vi "Code String Panel.vi"(11 "Code String":refnum<class "Code String LV.lvclass">) -> ()   [LabVIEW 2016, in "Code String LV.lvclass"]
doc: "Code String panel process.\n--------------------\nCopyright (c) 2019 Analog Devices, Inc. All rights reserved.\n\nRedistribution and use in source and binary forms, with or without modification,\nare permitted provided that the following conditions are met:\n - Redistributions of source code must retain the above copyright notice, this\n list of conditions and the following disclaimer.\n - Redistributions in binary form must reproduce the above copyright notice,\n this list of conditions and the following disclaimer in the documentation\n and/or other materials provided with the distribution.\n - Modified versions of the software must be conspicuously marked as such.\n - This software is licensed solely and exclusively for use with\n processors/products manufactured by or for Analog Devices, Inc.\n - This software may not be combined or merged with other code in any manner\n that would cause the software to become subject to terms and conditions\n which differ from those listed here.\n - Neither the name of Analog Devices, Inc. nor the names of its contributors\n may be used to endorse or promote products derived from this software\n without specific prior written permission.\n - The use of this software may or may not infringe the patent rights of one or\n more patent holders. This license does not release you from the requirement\n that you obtain separate licenses from these patent holders to use this\n software.\n\nTHIS SOFTWARE IS PROVIDED BY ANALOG DEVICES, INC. AND CONTRIBUTORS \"AS IS\" AND\nANY EXPRESS OR IMPLIED WARRANTIES, INCLUDING, BUT NOT LIMITED TO,\nNON-INFRINGEMENT, TITLE, MERCHANTABILITY AND FITNESS FOR A PARTICULAR PURPOSE\nARE DISCLAIMED. IN NO EVENT SHALL ANALOG DEVICES, INC. OR CONTRIBUTORS BE LIABLE\nFOR ANY DIRECT, INDIRECT, INCIDENTAL, SPECIAL, EXEMPLARY, PUNITIVE OR\nCONSEQUENTIAL DAMAGES (INCLUDING, BUT NOT LIMITED TO, DAMAGES ARISING OUT OF\nCLAIMS OF INTELLECTUAL PROPERTY RIGHTS INFRINGEMENT; PROCUREMENT OF SUBSTITUTE\nGOODS OR SERVICES; LOSS OF USE, DATA, OR PROFITS; OR BUSINESS INTERRUPTION)\nHOWEVER CAUSED AND ON ANY THEORY OF LIABILITY, WHETHER IN CONTRACT, STRICT\nLIABILITY, OR TORT (INCLUDING NEGLIGENCE OR OTHERWISE) ARISING IN ANY WAY OUT OF\nTHE USE OF THIS SOFTWARE, EVEN IF ADVISED OF THE POSSIBILITY OF SUCH DAMAGE.\n\n2019-01-10-7CBSD SLA"
uses:
  Code String LV.lvclass
  C:/Git/ipn_lv_dev/code-string/source/library/Code String/Code String/Code String.lvclass
  Code String/UI Logic/ASCII.ctl
  Code String/Events/Menu Item.ctl
  Suggestion Box/Suggestion Box.lvclass
  Suggestion Box/Events/Update Data.ctl
  <vilib>/Utility/miscctls.llb/LVPositionTypeDef.ctl
  <vilib>/Utility/miscctls.llb/LVSelectionTypeDef.ctl
  <vilib>/Utility/miscctls.llb/LVPointTypeDef.ctl
  <vilib>/Utility/miscctls.llb/LVRectTypeDef.ctl
  Suggestion Box/Suggestion Box.lvclass/Suggestion Box.ctl
  <vilib>/event_ctls.llb/lveventtype.ctl
  <vilib>/Utility/miscctls.llb/LVFontTypeDef.ctl
  Code String/State/Write Selected Text State.vi
  Code String/Properties/Read Completion.vi
  Code String/Properties/Read Editable.vi
  Code String/Properties/Write Completion.vi
  Code String/State/Write Text State.vi
  Code String/Properties/Read Active Ref.vi
  Code String/Properties/Read User Menu Items.vi
  Code String/Properties/Write User Menu Items.vi
  Code String/Properties/Read Rendezvous.vi
  Code String/Properties/Read User Events.vi
  Code String/Properties/Read Delimiter Pattern.vi
  <userlib>/_OpenG.lib/comparison/comparison.llb/String Changed__ogtk.vi
  Code String/Properties/Write Selected Line(s).vi
  Code String/Properties/Write # Selected Lines.vi
  Code String/Properties/Write Selected Token.vi
  Code String/Properties/Font Global.vi
  Code String/Properties/Write Active Ref.vi
  Code String/Properties/Read Selected Text.vi
  Code String/Properties/Read Text.vi
  <userlib>/_OpenG.lib/comparison/comparison.llb/U32 Changed__ogtk.vi
  Code String/Properties/Read Keywords.vi
  <userlib>/_OpenG.lib/comparison/comparison.llb/I32 Changed__ogtk.vi
  Code String/Code String.lvclass
panel:
  in  "Decoration":string
  in  "Line Numbers":i32(listbox)=-1
  out "String Indicator":string
  in  "String Control":string
  in  "Scrollbar":i32(c297)
  # "Copyright (c) 2019 Analog Devices, Inc.  All rights reserved.\n\nRedistribution and use in source and binary forms, with or without modification,\nare permitted provided that the following conditions are met:\n  - Redistributions of source code must retain the above copyright notice, this\n    list of conditions and the following disclaimer.\n  - Redistributions in binary form must reproduce the above copyright notice,\n    this list of conditions and the following disclaimer in the documentation\n    and/or other materials provided with the distribution.\n  - Modified versions of the software must be conspicuously marked as such.\n  - This software is licensed solely and exclusively for use with\n    processors/products manufactured by or for Analog Devices, Inc.\n  - This software may not be combined or merged with other code in any manner\n    that would cause the software to become subject to terms and conditions\n    which differ from those listed here.\n  - Neither the name of Analog Devices, Inc. nor the names of its contributors\n    may be used to endorse or promote products derived from this software\n    without specific prior written permission.\n  - The use of this software may or may not infringe the patent rights of one or\n    more patent holders.  This license does not release you from the requirement\n    that you obtain separate licenses from these patent holders to use this\n    software.\n\nTHIS SOFTWARE IS PROVIDED BY ANALOG DEVICES, INC. AND CONTRIBUTORS \"AS IS\" AND\nANY EXPRESS OR IMPLIED WARRANTIES, INCLUDING, BUT NOT LIMITED TO,\nNON-INFRINGEMENT, TITLE, MERCHANTABILITY AND FITNESS FOR A PARTICULAR PURPOSE\nARE DISCLAIMED. IN NO EVENT SHALL ANALOG DEVICES, INC. OR CONTRIBUTORS BE LIABLE\nFOR ANY DIRECT, INDIRECT, INCIDENTAL, SPECIAL, EXEMPLARY, PUNITIVE OR\nCONSEQUENTIAL DAMAGES (INCLUDING, BUT NOT LIMITED TO, DAMAGES ARISING OUT OF\nCLAIMS OF INTELLECTUAL PROPERTY RIGHTS INFRINGEMENT; PROCUREMENT OF SUBSTITUTE\nGOODS OR SERVICES; LOSS OF USE, DATA, OR PROFITS; OR BUSINESS INTERRUPTION)\nHOWEVER CAUSED AND ON ANY THEORY OF LIABILITY, WHETHER IN CONTRACT, STRICT\nLIABILITY, OR TORT (INCLUDING NEGLIGENCE OR OTHERWISE) ARISING IN ANY WAY OUT OF\nTHE USE OF THIS SOFTWARE, EVEN IF ADVISED OF THE POSSIBILITY OF SUCH DAMAGE.\n\n2019-01-10-7CBSD SLA"
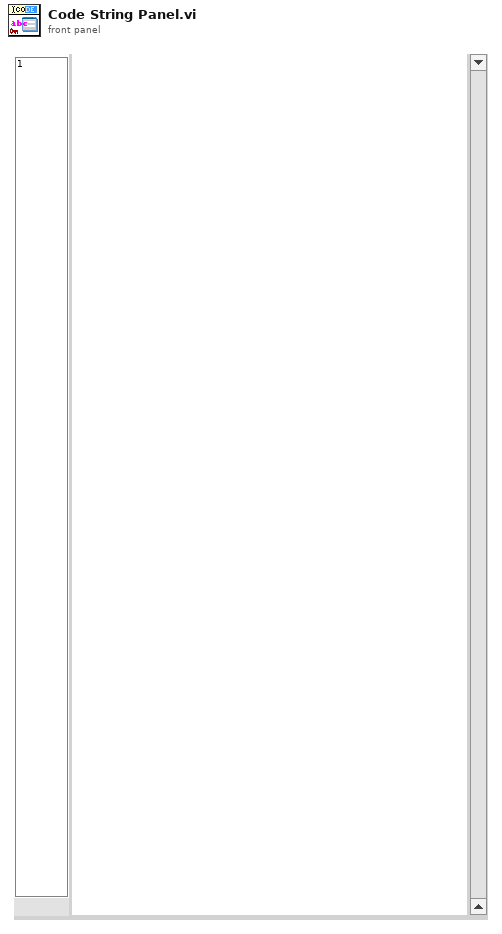
[diagram p1: front panel]
types:
  T1 = typedef "Code String.lvclass/ASCII.ctl" = enum8{"NUL", "SOH", "STX", "ETX", "EOT", "ENQ", "ACK", "BEL", "BS", "HT", "LF", "VT", "FF", "CR", "SO", "SI", "DLE", "DC1", "DC2", "DC3", "DC4", "NAK", "SYN", "ETB", "CAN", "EM", "SUB", "ESC", "FS", "GS", "RS", "US", "SP", "!", "\"", "#", "$", "%", "&", "'", "(", ")", "*", "+", ",", "- ", ".", "/", "0", "1", "2", "3", "4", "5", "6", "7", "8", "9", ":", ";", "<", "=", ">", "?", "@", "A", "B", "C", "D", "E", "F", "G", "H", "I", "J", "K", "L", "M", "N", "O", "P", "Q", "R", "S", "T", "U", "V", "W", "X", "Y", "Z", "[", "\\", "]", "^", "_", "`", "a", "b", "c", "d", "e", "f", "g", "h", "i", "j", "k", "l", "m", "n", "o", "p", "q", "r", "s", "t", "u", "v", "w", "x", "y", "z", "{", "|", "}", "~", "DEL"}
  T2 = typedef "Code String.lvclass/Menu Item.ctl" = cluster{"Item Path":string, "Visible?":bool, "Checked?":bool}
  T3 = enum32{"Invalid", "Standard", "Closed", "Hidden", "Minimized", "Maximized"}
  T4 = enum32{"invalid app kind", "Development System", "Run Time System", "Student Edition", "Embedded LabVIEW", "Evaluation", "Custom"}
  T5 = typedef "lveventtype.ctl" = enum32{"Null", "Timeout", "Annotation Menu Selection", "Annotation Menu Selection?", "App Instance Close", "App Instance Close?", "Autoscale Range Change", "Bookmark Info Change", "Cell Edit", "Cell Edit?", "Cursor Grab", "Cursor Grab?", "Cursor Menu Selection", "Cursor Menu Selection?", "Cursor Move", "Cursor Release", "Data Change", "Direction Change", "Display State Change", "Drag Ended", "Drag Enter", "Drag Leave", "Drag Over", "Drag Source Update", "Drag Starting", "Drag Starting?", "Drop", "Exec State Change", "Key Down", "Key Down?", "Key Repeat", "Key Repeat?", "Key Up", "Listbox Double Click", "Menu Activation?", "Menu Selection (App)", "Menu Selection? (App)", "Menu Selection (User)", "Mouse Down", "Mouse Down?", "Mouse Enter", "Mouse Leave", "Mouse Move", "Mouse Up", "Mouse Wheel", "NI Security User Change (App)", "Pane Size", "Panel Close", "Panel Close?", "Panel Resize", "Plot Attribute Change", "Scale Range Change", "Shortcut Menu Activation?", "Shortcut Menu Selection (App)", "Shortcut Menu Selection? (App)", "Shortcut Menu Selection (User)", "Tree Double Click", "Tree Drag", "Tree Drag?", "Tree Drop", "Tree Drop?", "Tree Item Close", "Tree Item Close?", "Tree Item Open", "Tree Item Open?", "User Event", "Value Change"}
  T6 = typedef "LVPointTypeDef.ctl" = cluster{"Horizontal":i16, "Vertical":i16}
  T7 = cluster{"Selection Start":i32, "Selection End":i32}
  T8 = typedef "LVPositionTypeDef.ctl" = cluster{"Left":i32, "Top":i32}
  T9 = typedef "LVFontTypeDef.ctl" = cluster{"Font Name":string, "Size":u16, "Bold":bool, "Italic":bool, "Underline":bool, "Strikeout":bool, "Color":u32}
  T10 = typedef "LVPoint32TypeDef.ctl" = cluster{"Horizontal":i32, "Vertical":i32}
  T11 = typedef "Suggestion Box.lvclass/Update Data.ctl" = cluster{"Query":string, "Keywords":string[], "Position":T8}
  T12 = typedef "LVSelectionTypeDef.ctl" = cluster{"Selection Start":u32, "Selection End":u32}
  T13 = typedef "LVRectTypeDef.ctl" = cluster{"Left":i16, "Top":i16, "Right":i16, "Bottom":i16}
  T14 = cluster{"Core":cluster{"Current VI Reference":refnum<vi>, "Close Panel on Exit?":bool}, "T":i32, "Panes":refnum<vi>[], "Strings":refnum<vi>[], "Line #":refnum<vi>, "Scrollbar":refnum<vi>, "Suggestions":cluster{"Suggestion Box":refnum<class "Suggestion Box.lvclass">, "Visible?":bool, "Display Limit":i32, "Update Data":T11, "Selected":string, "Location":T12, "Delta?":bool}, "Mouse Down":cluster{"?":bool, "Offset":T6, "Bounds":T13}}
  T15 = typedef "eventvkey.ctl" = enum16{"ASCII", "Enter", "Return", "Shift", "Ctrl", "Alt", "Cmd", "Opt", "Caps", "NumLock", "Clear", "Break", "Up", "Down", "Left", "Right", "Insert", "Delete", "Home", "End", "PageUp", "PageDown", "Escape", "Help", "Pause", "ScrollLock", "F1", "F2", "F3", "F4", "F5", "F6", "F7", "F8", "F9", "F10", "F11", "F12", "F13", "F14", "F15", "F16", "F17", "F18", "F19", "F20", "F21", "F22", "F23", "F24", "Play", "VolumeUp", "VolumeDown", "Mute", "Two Byte Char"}
  T16 = typedef "Rendezvous RefNum" = refnum<k1>
  T17 = cluster{"Suggestion Box":refnum<class "Suggestion Box.lvclass">, "Visible?":bool, "Display Limit":i32, "Update Data":T11, "Selected":string, "Location":T12, "Delta?":bool}
  T18 = cluster{"Current VI Reference":refnum<vi>, "Close Panel on Exit?":bool}
  T19 = typedef "Code String.lvclass/User Events.ctl" = cluster{"Exit":refnum<user-event>, "Editable Changed":refnum<user-event>, "Font Size Changed":refnum<user-event>, "Font Color Changed":refnum<user-event>, "Text Selection Start Changed":refnum<user-event>, "Text Selection End Changed":refnum<user-event>, "Scroll Position Changed":refnum<user-event>, "Shortcut Menu Item":refnum<user-event>, "Text":refnum<user-event>, "Selected Text":refnum<user-event>}
  T20 = typedef "Suggestion Box.lvclass/Public Events.ctl" = cluster{"Suggestion Selected":refnum<user-event>}
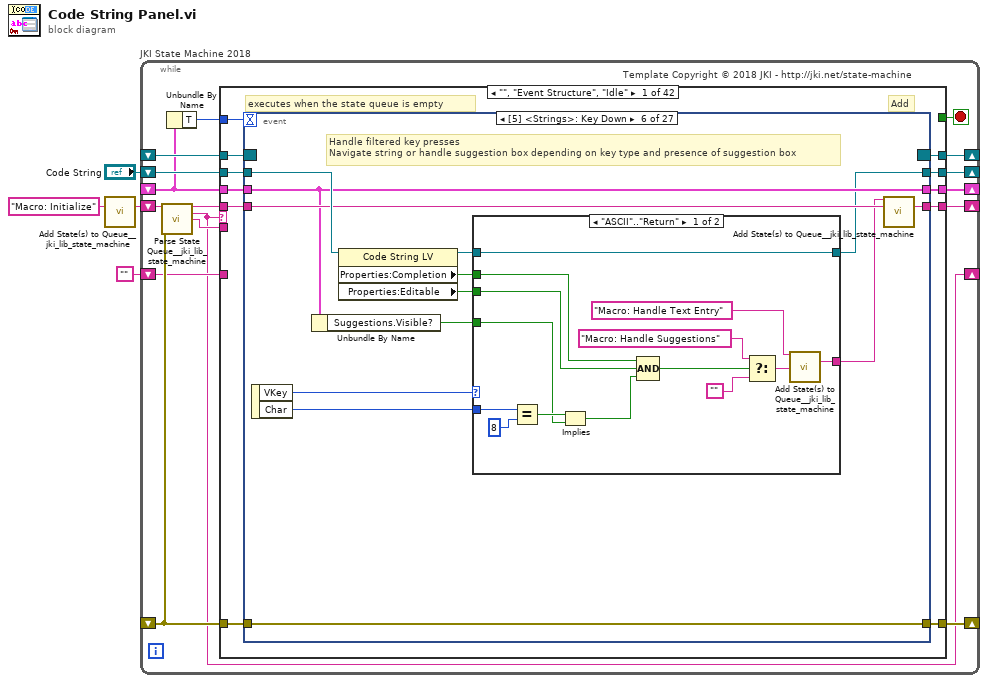
[diagram p0: block diagram]
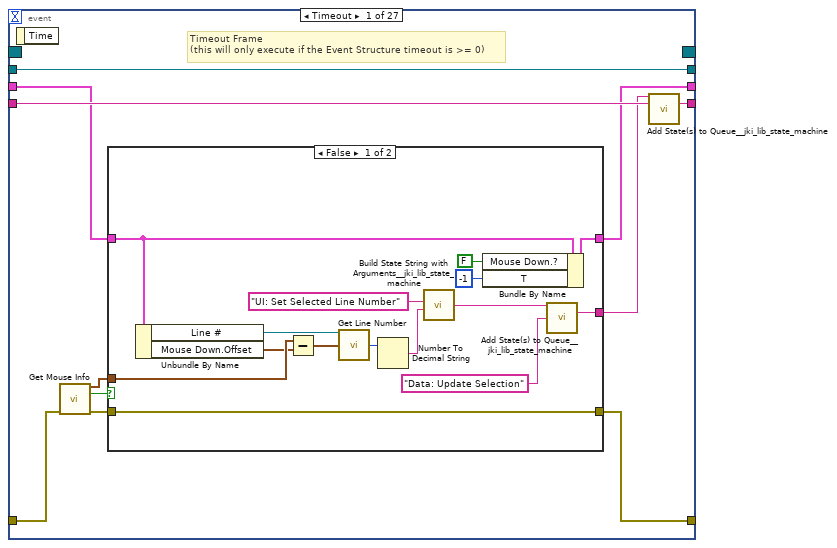
[diagram p2: hidden frame]
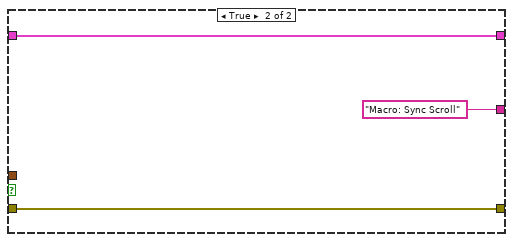
[diagram p3: hidden frame]
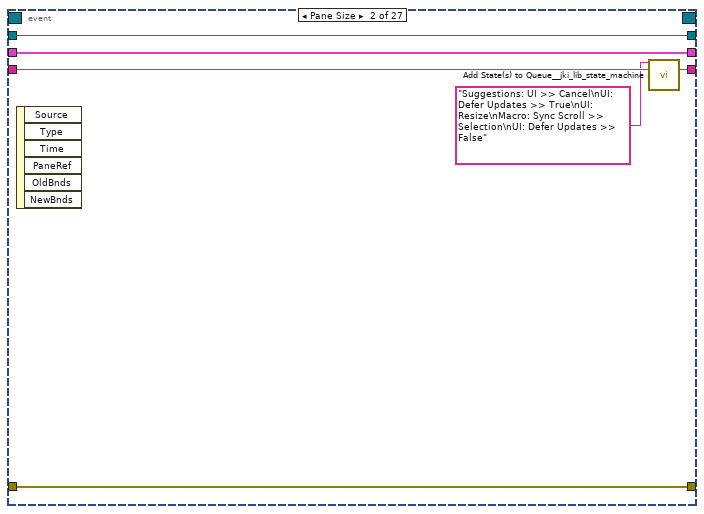
[diagram p4: hidden frame]
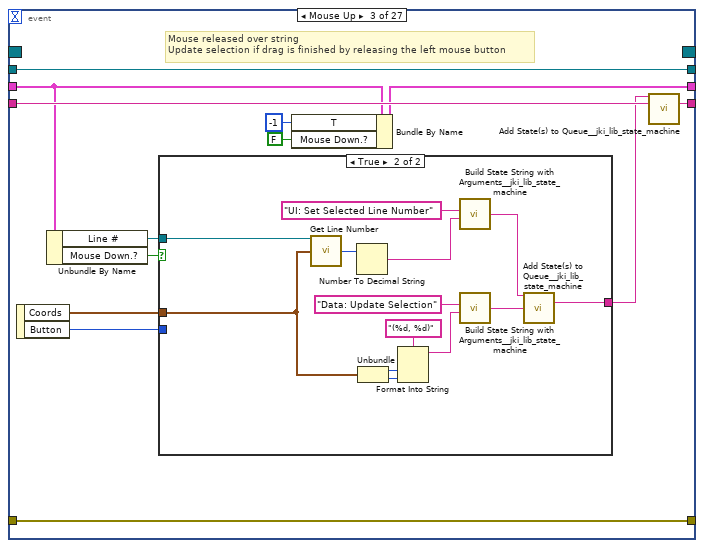
[diagram p5: hidden frame]
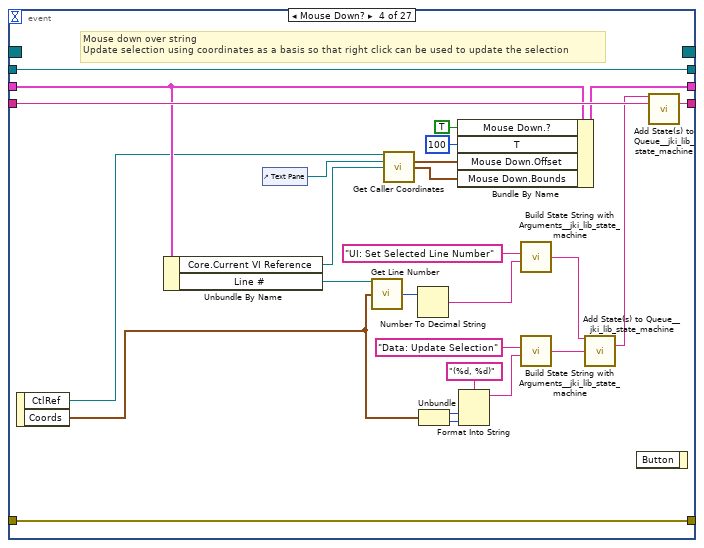
[diagram p7: hidden frame]
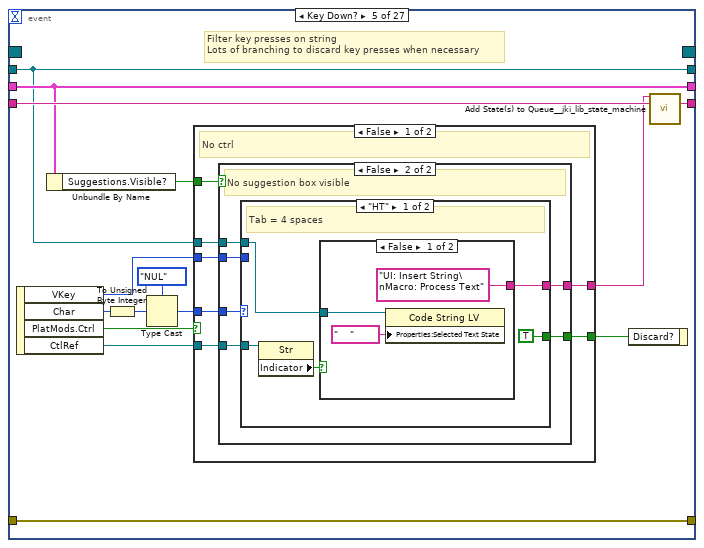
[diagram p8: hidden frame]
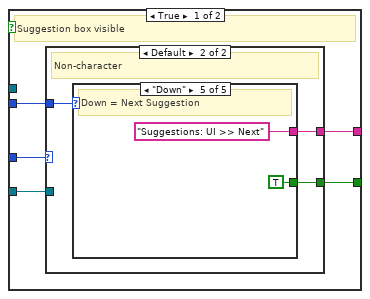
[diagram p9: hidden frame]
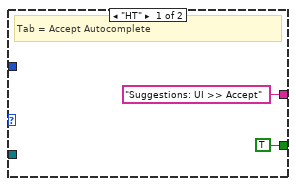
[diagram p10: hidden frame]
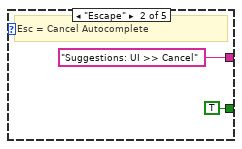
[diagram p12: hidden frame]
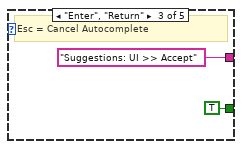
[diagram p13: hidden frame]
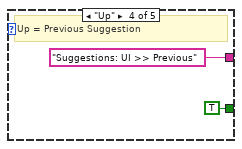
[diagram p14: hidden frame]
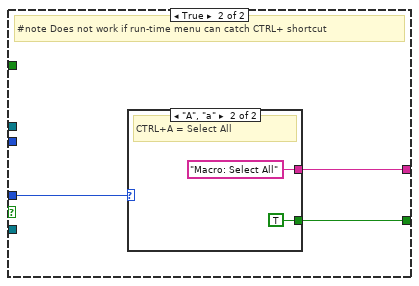
[diagram p17: hidden frame]
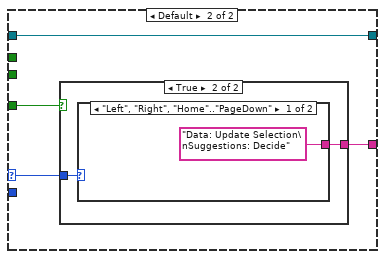
[diagram p19: hidden frame]
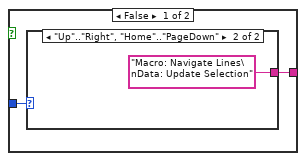
[diagram p20: hidden frame]
diagram:
  n1 = call <vilib>:"Add State(s) to Queue__jki_lib_state_machine.vi"("State(s) in (\"\")"="Macro: Initialize") -> ("States Out"=w4:string)  [unwired: 14 in]
  n2 = while "JKI State Machine 2018" {
    shift-right: [w15] -> _
    shift-left: _ -> [w9]
    shift-right: [w17] -> _
    shift-left: _ -> [w14]
    shift-right: [w8] -> _
    shift-left: w4 -> [w18]
    shift-right: [w13] -> _
    shift-left: "Code String" -> [w12]
    shift-right: [w11] -> _
    shift-left: _ -> [w10]
    shift-right: [w6] -> _
    shift-left: "" -> [w7]
    stop <- w16 stop-if-true
    # "Template Copyright © 2018 JKI - http://jki.net/state-machine"
    n3 = call <vilib>:"Parse State Queue__jki_lib_state_machine.vi"("State Queue"=w18, "Error In (no error)"=w14) -> ("Remaining States"=w20:string, "Current State"=w6:string, "Arguments"=w19:string)  [unwired: 11 in]
    n4 = Unbundle By Name(w9) -> ("T"=w5:i32)
    n5 = case shown="\"\", \"Event Structure\", \"Idle\"" w6 {
      selector: w6 -> [_ _ w480 _ _ _ _ _ _ _ _ _ _ _ _ _ _ _ _ _ _ _ _ _ _ _ _ _ _ _ _ _ _ _ _ _ _ _ _ _ _ _]
      tunnel: w20 -> [w31 w477 w484 w505 w514 w522 w529 w535 w557 w570 w591 w627 w642 w648 w674 w692 w705 w784 w801 w816 w838 w857 w868 w920 w935 w951 w978 w1000 w1024 w1039 w1057 w1073 w1082 w1152 w1159 w1179 w1192 w1199 w1206 w1217 w1235 w1256]
      tunnel: w19 -> [_ _ _ _ _ _ _ _ _ _ w582 _ _ _ _ w687 w699 w780 _ _ w826 _ w864 _ w927 w946 _ w997 _ _ _ _ w1076 _ _ w1172 w1183 _ _ _ w1224 w1242]
      tunnel: w9 -> [w29 w474 w482 w498 w512 w519 w527 w532 _ w567 w588 w625 w637 w645 w650 w690 w701 w779 w787 w815 w834 w849 w859 w910 w929 w944 w967 w992 w1021 w1032 w1041 w1065 w1081 w1149 w1156 w1176 w1189 w1196 w1203 w1220 w1238 w1253]
      tunnel: [w28 w475 w486 w502 w508 errorcluster {"status"=FALSE, "code"=0, "source"=""} ("error out") w526 w533 w555 w568 w581 w617 w638 w646 w666 w688 w702 w771 w799 w810 w836 w851 w865 w918 w933 w949 w976 w993 w1022 w1035 w1045 w1071 w1077 w1150 w1157 w1177 w1190 w1197 w1204 w1221 w1239 w1254] -> w17
      tunnel: w14 -> [w27 w475 w485 w502 w509 w518 w526 w533 w555 w563 w589 w618 w639 w646 w666 w689 w703 w774 w799 w811 w836 w852 w865 w918 w933 w949 w976 w994 w1022 w1035 w1046 w1071 w1078 w1150 w1157 w1177 w1190 w1197 w1204 w1221 w1239 w1254]
      tunnel: [w30 w476 w483 w504 w513 w521 w528 w534 w557 w569 w590 w626 w641 w647 w673 w691 w704 w783 w800 w816 w837 w856 w868 w919 w934 w950 w977 w999 w1023 w1038 w1056 w1072 w1082 w1151 w1158 w1178 w1191 w1198 w1205 w1222 w1240 w1255] -> w8
      tunnel: [_ _ _ _ _ _ TRUE _ _ _ _ _ _ _ _ _ _ _ _ _ _ _ _ _ _ _ _ _ _ _ _ _ _ _ _ _ _ _ _ _ _ _] -> w16
      tunnel: [w26 w474 w482 w503 w512 w519 w527 w532 w556 w567 w575 w625 w637 w645 w650 w690 w701 w779 w787 w815 w834 w849 w859 w910 w929 w944 w967 w992 w1021 w1036 w1053 w1065 w1079 w1149 w1156 w1176 w1189 w1196 w1203 w1220 w1238 w1253] -> w15
      tunnel: w5 -> [w25 _ _ _ _ _ _ _ _ _ _ _ _ _ _ _ _ _ _ _ _ _ _ _ _ _ _ _ _ _ _ _ _ _ _ _ _ _ _ _ _ _]
      tunnel: [w22 w473 w479 w492 w507 w516 w524 w531 w543 w558 w579 w621 w636 w644 w656 w686 w698 w782 w788 w814 w829 w853 w861 w912 w930 w947 w973 w995 w1020 w1034 w1054 w1068 w1074 w1148 w1154 w1170 w1188 w1195 w1202 w1219 w1237 w1247] -> w13
      tunnel: w12 -> [w23 w473 w479 w492 w507 w516 w524 w531 w543 w558 w586 w622 w636 w644 w656 w686 w698 w782 w788 w814 w828 w854 w866 w912 w930 w947 w973 w995 w1020 w1034 w1054 w1068 w1075 w1148 w1154 w1170 w1188 w1195 w1202 w1219 w1237 w1247]
      tunnel: [w24 w472 w478 w491 w511 w515 w523 w530 w553 w562 w587 w619 w634 w643 w672 w685 w697 w781 w798 w812 w835 w855 w867 w917 w932 w948 w975 w998 w1019 w1037 w1055 w1070 w1080 w1147 w1153 w1175 w1187 w1194 w1201 w1218 w1236 w1246] -> w11
      tunnel: w10 -> [w21 w472 w478 w491 w511 w515 w523 w530 w553 _ w587 w620 w634 w643 w672 w685 w697 w781 w798 w813 w835 w855 w867 w917 w932 w948 w975 w998 w1019 w1037 w1055 w1070 w1080 w1147 w1153 w1175 w1187 w1194 w1201 w1218 w1236 w1246]
      tunnel: w7 -> [_ _ _ _ _ _ _ _ _ _ _ _ _ _ _ _ _ _ _ _ _ _ _ _ _ _ _ _ _ _ _ _ _ _ _ _ _ _ _ w1207 w1226 _]
      frame "", "Event Structure", "Idle" {
        # "Add"
        # "executes when the state queue is empty"
        n6 = event shown="[5] <Strings>: Key Down" {
          selector: w21 -> [_ _ _ _ _ _ _ _ _ _ _ _ _ _ _ _ _ _ _ _ _ _ _ _ _ _ _]
          dyn-events: [_ _ _ _ _ _ _ _ _ _ _ _ _ _ _ _ _ _ _ _ _ _ _ _ _ _ _] -> w24
          timeout: w25 -> [_ _ _ _ _ _ _ _ _ _ _ _ _ _ _ _ _ _ _ _ _ _ _ _ _ _ _]
          tunnel: w31 -> [w42 w62 w77 w116 w126 w187 w220 w228 w240 w251 w296 w305 w313 w329 w340 w366 w371 w380 w392 w404 w416 w422 w428 w442 w447 w461 w471]
          tunnel: [w41 w63 w78 w117 w127 w188 w220 w229 w241 w252 w296 w306 w313 w330 w341 w367 w372 w381 w393 w405 w417 w423 w429 w442 w448 w462 w470] -> w30
          tunnel: w29 -> [w33 w66 w73 w100 w124 w183 w219 w225 w244 w254 w294 w303 w311 w322 w348 w369 w375 w384 w396 w408 w419 w425 w431 w434 w452 w464 w468]
          tunnel: [w38 w64 w79 w118 w119 w189 w217 w230 w242 w249 w292 w307 w312 w331 w343 w365 w373 w382 w394 w406 w418 w424 w430 w440 w450 w454 w469] -> w28
          tunnel: w27 -> [w40 w64 w79 w118 w119 w189 w217 w230 w242 w253 w289 w307 w312 w331 w346 w365 w373 w382 w394 w406 w418 w424 w430 w440 w450 w454 w469]
          tunnel: [w32 w66 w70 w108 w124 w183 w219 w225 w244 w254 w294 w303 w311 w322 w348 w369 w375 w384 w396 w408 w419 w425 w431 w434 w449 w464 w468] -> w26
          tunnel: w23 -> [w36 w65 w74 w93 w120 w190 w218 w223 w243 w250 w287 w304 w310 w324 w333 w368 w374 w383 w395 w407 w415 w420 w426 w441 w451 w463 w465]
          tunnel: [w36 w65 w74 w93 w120 w179 w218 w223 w243 w247 w285 w304 w310 w324 w333 w368 w374 w383 w395 w407 w415 w420 w426 w439 w451 w463 w465] -> w22
          event Timeout {
            # "Timeout Frame\n(this will only execute if the Event Structure timeout is >= 0)"
            n7 = event-data() -> ()  [unwired: 1 in, 1 out]
            n8 = call "Get Mouse Info.vi"("error in (no error)"=w40) -> ("Coordinates"=w35:T10, "Left Mouse Button?"=w37:bool, "error out"=w39:errorcluster)  [unwired: 11 in, 1 out]
            n9 = case shown="False" w37 {
              tunnel: w39 -> [w57 w58]
              tunnel: [w57 w58] -> w38
              tunnel: w35 -> [w56 _]
              tunnel: [w45 "Macro: Sync Scroll"] -> w34
              tunnel: w33 -> [w55 w60]
              tunnel: [w43 w60] -> w32
              frame False {
                n10 = Unbundle By Name(w55) -> ("Line #"=w54:refnum<vi>, "Mouse Down.Offset"=w47:T6)
                n11 = Subtract(x=w56, y=w47) -> (x-y=w48:T10)
                n12 = call "Get Line Number.vi"("Line Numbers in"=w54, "Coords"=w48) -> ("Row"=w51:i32)  [unwired: 12 in, 1 out]
                n13 = Number To Decimal String(number=w51) -> (decimal integer string=w52:string)  [unwired: 1 in]
                n14 = call <vilib>:"Build State String with Arguments__jki_lib_state_machine.vi"("Arguments (\"\")"=w52, "State"="UI: Set Selected Line Number") -> ("State with Arguments"=w46:string)  [unwired: 4 in]
                n15 = Bundle By Name(cluster=w55, "Mouse Down.?"=FALSE ("Mouse Down?"), "T"=-1) -> (w43:T14)
                n16 = call <vilib>:"Add State(s) to Queue__jki_lib_state_machine.vi"("State(s) in Front (\"\")"=w46, "State(s) at Back (\"\")"="Data: Update Selection") -> ("States Out"=w45:string)  [unwired: 13 in]
              }
              frame True {
              }
            }
            n17 = call <vilib>:"Add State(s) to Queue__jki_lib_state_machine.vi"("State(s) in Front (\"\")"=w34, "State(s) in (\"\")"=w42) -> ("States Out"=w41:string)  [unwired: 13 in]
          }
          event Pane Size {
            n18 = event-data() -> ()  [unwired: 1 in, 6 out]
            n19 = call <vilib>:"Add State(s) to Queue__jki_lib_state_machine.vi"("State(s) in Front (\"\")"="Suggestions: UI >> Cancel\nUI: Defer Updates >> True\nUI: Resize\nMacro: Sync Scroll >> Selection\nUI: Defer Updates >> False", "State(s) in (\"\")"=w62) -> ("States Out"=w63:string)  [unwired: 13 in]
          }
          event Mouse Up {
            # "Mouse released over string\nUpdate selection if drag is finished by releasing the left mouse button"
            n20 = event-data() -> ("Coords"=w71:T10, "Button"=w76:u16)  [unwired: 1 in]
            n21 = Unbundle By Name(w73) -> ("Line #"=w68:refnum<vi>, "Mouse Down.?"=w72:bool)
            n22 = case shown="True" w72 {
              tunnel: w76 -> [_ _]
              tunnel: [_ w92] -> w75
              tunnel: w71 -> [_ w91]
              tunnel: w68 -> [_ w90]
              frame False {
              }
              frame True {
                n23 = call "Get Line Number.vi"("Line Numbers in"=w90, "Coords"=w91) -> ("Row"=w83:i32)  [unwired: 12 in, 1 out]
                n24 = Number To Decimal String(number=w83) -> (decimal integer string=w84:string)  [unwired: 1 in]
                n25 = Unbundle(w91) -> ("Horizontal"=w89:i32, "Vertical"=w88:i32)
                n26 = Format Into String(format string="(%d, %d)", w89, w88) -> (resulting string=w86:string)  [unwired: 2 in, 1 out]
                n27 = call <vilib>:"Build State String with Arguments__jki_lib_state_machine.vi"("Arguments (\"\")"=w84, "State"="UI: Set Selected Line Number") -> ("State with Arguments"=w82:string)  [unwired: 4 in]
                n28 = call <vilib>:"Build State String with Arguments__jki_lib_state_machine.vi"("Arguments (\"\")"=w86, "State"="Data: Update Selection") -> ("State with Arguments"=w80:string)  [unwired: 4 in]
                n29 = call <vilib>:"Add State(s) to Queue__jki_lib_state_machine.vi"("State(s) in Front (\"\")"=w82, "State(s) in (\"\")"=w80) -> ("States Out"=w92:string)  [unwired: 13 in]
              }
            }
            n30 = Bundle By Name(cluster=w73, "T"=-1, "Mouse Down.?"=FALSE) -> (w70:T14)
            n31 = call <vilib>:"Add State(s) to Queue__jki_lib_state_machine.vi"("State(s) in Front (\"\")"=w75, "State(s) in (\"\")"=w77) -> ("States Out"=w78:string)  [unwired: 13 in]
          }
          event Mouse Down? {
            # "Mouse down over string\nUpdate selection using coordinates as a basis so that right click can be used to update the selection"
            n32 = event-data() -> ("CtlRef"=w94:refnum<vi>, "Coords"=w105:T10)  [unwired: 1 in]
            n33 = Unbundle By Name(w100) -> ("Core.Current VI Reference"=w97:refnum<vi>, "Line #"=w106:refnum<vi>)
            n34 = control-ref of="Text Pane"() -> (w101:refnum<vi>)
            n35 = call "Get Line Number.vi"("Line Numbers in"=w106, "Coords"=w105) -> ("Row"=w104:i32)  [unwired: 12 in, 1 out]
            n36 = call "Get Caller Coordinates.vi"("Control in"=w94, "Pane"=w101, "VI"=w97) -> ("Control Position"=w99:T6, "Control Bounds"=w98:T13)  [unwired: 9 in, 2 out]
            n37 = Number To Decimal String(number=w104) -> (decimal integer string=w109:string)  [unwired: 1 in]
            n38 = Unbundle(w105) -> ("Horizontal"=w115:i32, "Vertical"=w114:i32)
            n39 = Bundle By Name(cluster=w100, "Mouse Down.?"=TRUE ("Mouse Down?"), "T"=100, "Mouse Down.Offset"=w99, "Mouse Down.Bounds"=w98) -> (w108:T14)
            n40 = Format Into String(format string="(%d, %d)", w115, w114) -> (resulting string=w112:string)  [unwired: 2 in, 1 out]
            n41 = call <vilib>:"Build State String with Arguments__jki_lib_state_machine.vi"("Arguments (\"\")"=w109, "State"="UI: Set Selected Line Number") -> ("State with Arguments"=w103:string)  [unwired: 4 in]
            n42 = call <vilib>:"Build State String with Arguments__jki_lib_state_machine.vi"("Arguments (\"\")"=w112, "State"="Data: Update Selection") -> ("State with Arguments"=w95:string)  [unwired: 4 in]
            n43 = call <vilib>:"Add State(s) to Queue__jki_lib_state_machine.vi"("State(s) in Front (\"\")"=w103, "State(s) in (\"\")"=w95) -> ("States Out"=w111:string)  [unwired: 13 in]
            n44 = event-data() -> ()  [unwired: 2 in, 1 out]
            n45 = call <vilib>:"Add State(s) to Queue__jki_lib_state_machine.vi"("State(s) in Front (\"\")"=w111, "State(s) in (\"\")"=w116) -> ("States Out"=w117:string)  [unwired: 13 in]
          }
          event Key Down? {
            # "Filter key presses on string\nLots of branching to discard key presses when necessary"
            n46 = event-data() -> ("VKey"=w125:T15, "Char"=w132:i16, "PlatMods.Ctrl"=w133:bool, "CtlRef"=w128:refnum<vi>)  [unwired: 1 in]
            n47 = Unbundle By Name(w124) -> ("Suggestions.Visible?"=w123:bool)
            n48 = To Unsigned Byte Integer(number=w132) -> (unsigned 8bit integer=w129:u8)
            n49 = Type Cast(type=ASCII."NUL" ("ASCII"), x=w129) -> (*(type *) &x=w130:T1)
            n50 = case shown="False" w133 {
              tunnel: [w139 w175] -> w121
              tunnel: w130 -> [w140 w174]
              tunnel: w128 -> [w138 _]
              tunnel: [w137 w173] -> w122
              tunnel: w125 -> [w136 _]
              tunnel: w123 -> [w135 _]
              tunnel: w120 -> [w134 _]
              frame False {
                # "No ctrl"
                n51 = case shown="False" w135 {
                  tunnel: w140 -> [w145 w164]
                  tunnel: [w144 w163] -> w139
                  tunnel: w138 -> [w143 w162]
                  tunnel: [w142 w159] -> w137
                  tunnel: w136 -> [w141 w161]
                  tunnel: w134 -> [_ w160]
                  frame True {
                    # "Suggestion box visible"
                    n52 = case shown="Default" w145 {
                      tunnel: [TRUE w150] -> w144
                      tunnel: w143 -> [_ _]
                      tunnel: ["Suggestions: UI >> Accept" w148] -> w142
                      tunnel: w141 -> [_ w149]
                      frame "HT" {
                        # "Tab = Accept Autocomplete"
                      }
                      frame Default {
                        # "Non-character"
                        n53 = case shown="\"Down\"" w149 {
                          tunnel: [_ TRUE TRUE TRUE TRUE] -> w150
                          tunnel: [_ "Suggestions: UI >> Cancel" "Suggestions: UI >> Accept" "Suggestions: UI >> Previous" "Suggestions: UI >> Next"] -> w148
                          frame Default {
                          }
                          frame "Escape" {
                            # "Esc = Cancel Autocomplete"
                          }
                          frame "Enter", "Return" {
                            # "Esc = Cancel Autocomplete"
                          }
                          frame "Up" {
                            # "Up = Previous Suggestion"
                          }
                          frame "Down" {
                            # "Down = Next Suggestion"
                          }
                        }
                      }
                    }
                  }
                  frame False {
                    # "No suggestion box visible"
                    n54 = case shown="\"HT\"" w164 {
                      tunnel: [TRUE _] -> w163
                      tunnel: w162 -> [w168 _]
                      tunnel: w161 -> [_ _]
                      tunnel: w160 -> [w166 _]
                      tunnel: [w165 _] -> w159
                      frame "HT" {
                        # "Tab = 4 spaces"
                        n55 = property class="Str"(reference=w168) -> ("Indicator"=w167:bool)  [unwired: 1 in, 2 out]
                        n56 = case shown="False" w167 {
                          tunnel: w166 -> [w171 _]
                          tunnel: ["UI: Insert String\nMacro: Process Text" _] -> w165
                          frame False {
                            n57 = property class="Code String LV"(reference=w171, "Properties:Selected Text State"="    " ("string")) -> ()  [unwired: 1 in, 2 out]
                          }
                          frame True {
                          }
                        }
                      }
                      frame Default {
                      }
                    }
                  }
                }
              }
              frame True {
                # "#note Does not work if run-time menu can catch CTRL+ shortcut"
                n58 = case shown="\"A\", \"a\"" w174 {
                  tunnel: [_ TRUE] -> w175
                  tunnel: [_ "Macro: Select All"] -> w173
                  frame Default {
                  }
                  frame "A", "a" {
                    # "CTRL+A = Select All"
                  }
                }
              }
            }
            n59 = event-data("Discard?"=w121) -> ()  [unwired: 1 in, 1 out]
            n60 = call <vilib>:"Add State(s) to Queue__jki_lib_state_machine.vi"("State(s) in Front (\"\")"=w122, "State(s) in (\"\")"=w126) -> ("States Out"=w127:string)  [unwired: 13 in]
          }
          event Key Down {
            # "Handle filtered key presses\nNavigate string or handle suggestion box depending on key type and presence of suggestion box"
            n61 = event-data() -> ("VKey"=w185:T15, "Char"=w178:i16)  [unwired: 1 in]
            n62 = Unbundle By Name(w183) -> ("Suggestions.Visible?"=w182:bool)
            n63 = property class="Code String LV"(reference=w190) -> (reference out=w180:refnum<class "Code String LV.lvclass">, "Properties:Completion"=w184:bool, "Properties:Editable"=w181:bool)  [unwired: 1 in, 1 out]
            n64 = case shown="\"ASCII\"..\"Return\"" w185 {
              selector: w185 -> [_ w208]
              tunnel: [w200 w207] -> w186
              tunnel: w184 -> [w204 _]
              tunnel: w182 -> [w192 w206]
              tunnel: w181 -> [w203 _]
              tunnel: w180 -> [w199 w205]
              tunnel: [w199 w205] -> w179
              tunnel: w178 -> [w196 _]
              frame "ASCII".."Return" {
                n65 = Equal?(x=w196, y=i16 8) -> (x = y?=w193:bool)
                n66 = Implies(1:w192, 2:w193) -> (0:w191:bool)
                n67 = Compound Arithmetic op=AND(w204, w203, w191) -> (w201:bool)
                n68 = Select(t="Macro: Handle Suggestions", s=w201, f="") -> (s? t:f=w197:string)
                n69 = call <vilib>:"Add State(s) to Queue__jki_lib_state_machine.vi"("State(s) in Front (\"\")"="Macro: Handle Text Entry", "State(s) at Back (\"\")"=w197) -> ("States Out"=w200:string)  [unwired: 13 in]
              }
              frame Default {
                n70 = case shown="True" w206 {
                  tunnel: w208 -> [w209 w213]
                  tunnel: [w210 w212] -> w207
                  frame False {
                    n71 = case shown="\"Up\"..\"Right\", \"Home\"..\"PageDown\"" w209 {
                      tunnel: [_ "Macro: Navigate Lines\nData: Update Selection"] -> w210
                      frame Default {
                      }
                      frame "Up".."Right", "Home".."PageDown" {
                      }
                    }
                  }
                  frame True {
                    n72 = case shown="\"Left\", \"Right\", \"Home\"..\"PageDown\"" w213 {
                      tunnel: ["Data: Update Selection\nSuggestions: Decide" _] -> w212
                      frame "Left", "Right", "Home".."PageDown" {
                      }
                      frame Default {
                      }
                    }
                  }
                }
              }
            }
            n73 = call <vilib>:"Add State(s) to Queue__jki_lib_state_machine.vi"("State(s) in Front (\"\")"=w186, "State(s) in (\"\")"=w187) -> ("States Out"=w188:string)  [unwired: 13 in]
          }
          event event type 1.0.x8000000b {
            # "Filter key repeats\nDiscard repeats that will edit the text due to glitching"
            n74 = event-data() -> ("VKey"=w216:T15)  [unwired: 1 in]
            n75 = case shown="\"ASCII\"..\"Return\", \"Delete\"" w216 {
              tunnel: [FALSE FALSE] -> w215
              frame Default {
              }
              frame "ASCII".."Return", "Delete" {
              }
            }
            n76 = event-data("Discard?"=w215) -> ()  [unwired: 1 in, 1 out]
          }
          event Key Repeat {
            # "Handle filtered key repeats\nNavigate string"
            n77 = event-data() -> ("VKey"=w226:T15)  [unwired: 1 in]
            n78 = Unbundle By Name(w225) -> ("Suggestions.Visible?"=w224:bool)
            n79 = case shown="False" w224 {
              tunnel: [w232 w237] -> w227
              tunnel: w226 -> [w231 w236]
              frame True {
                n80 = case shown="\"Left\", \"Right\", \"Home\"..\"PageDown\"" w231 {
                  tunnel: ["Suggestions: UI >> Previous" "Suggestions: UI >> Next" "Data: Update Selection\nSuggestions: Decide" _] -> w232
                  frame "Up" {
                  }
                  frame "Down" {
                  }
                  frame "Left", "Right", "Home".."PageDown" {
                  }
                  frame Default {
                  }
                }
              }
              frame False {
                n81 = case shown="\"Up\"..\"Right\", \"Home\"..\"PageDown\"" w236 {
                  tunnel: [_ "Macro: Navigate Lines\nData: Update Selection"] -> w237
                  frame Default {
                  }
                  frame "Up".."Right", "Home".."PageDown" {
                  }
                }
              }
            }
            n82 = call <vilib>:"Add State(s) to Queue__jki_lib_state_machine.vi"("State(s) in Front (\"\")"=w227, "State(s) in (\"\")"=w228) -> ("States Out"=w229:string)  [unwired: 13 in]
          }
          event Value Change {
            # "Handle value change event\ne.g. CTRL+X, CTRL+V. Should be flushed for key down operations"
            n83 = event-data() -> ()  [unwired: 1 in, 6 out]
            n84 = call <vilib>:"Add State(s) to Queue__jki_lib_state_machine.vi"("State(s) in Front (\"\")"="Macro: Handle Text Entry", "State(s) in (\"\")"=w240) -> ("States Out"=w241:string)  [unwired: 13 in]
          }
          event Shortcut Menu Selection (User) {
            # "Shortcut menu item selected\nHandle built-in menu options and broadcast event"
            n85 = event-data() -> ("ItemPath"=w245:string)  [unwired: 1 in]
            n86 = case shown="\"PASTE\"" w245 {
              tunnel: w250 -> [w255 w260 w262 w266 w270 w277 w283]
              tunnel: [w255 w256 w262 w265 w269 w273 w280] -> w248
              tunnel: [_ _ "Macro: Select All" "Macro: Process Text" _ "Macro: Process Text" "Macro: Process Text"] -> w246
              frame Default {
                # "No handling for other menu selections"
              }
              frame "AUTOCOMPLETE" {
                # "Toggle completion setting"
                n87 = property class="Code String LV"(reference=w260) -> (reference out=w259:refnum<class "Code String LV.lvclass">, "Properties:Completion"=w258:bool)  [unwired: 1 in, 1 out]
                n88 = Not(x=w258) -> (.not. x?=w257:bool)
                n89 = property class="Code String LV"(reference=w259, "Properties:Completion"=w257) -> (reference out=w256:refnum<class "Code String LV.lvclass">)  [unwired: 1 in, 1 out]
              }
              frame "SELECT ALL" {
                # "Select  all of the text in the code string"
              }
              frame "DELETE" {
                # "Set the value to an empty string"
                n90 = property class="Code String LV"(reference=w266, "Properties:Text State"="") -> (reference out=w265:refnum<class "Code String LV.lvclass">)  [unwired: 1 in, 1 out]
              }
              frame "COPY" {
                # "Copies the active text selection to the clipboard"
                n91 = property class="Code String LV"(reference=w270) -> (reference out=w269:refnum<class "Code String LV.lvclass">, "Properties:Active Ref"=w268:refnum<vi>)  [unwired: 1 in, 1 out]
                n92 = call "Copy String Selection.vi"("String in"=w268, "Cut? (F)"=FALSE) -> ()  [unwired: 10 in, 4 out]
              }
              frame "CUT" {
                # "Cuts the active text selection to the clipboard"
                n93 = property class="Code String LV"(reference=w277) -> (reference out=w276:refnum<class "Code String LV.lvclass">, "Properties:Active Ref"=w275:refnum<vi>)  [unwired: 1 in, 1 out]
                n94 = call "Copy String Selection.vi"("String in"=w275, "Cut? (F)"=TRUE) -> ("Result"=w271:string)  [unwired: 10 in, 3 out]
                n95 = property class="Code String LV"(reference=w276, "Properties:Text State"=w271) -> (reference out=w273:refnum<class "Code String LV.lvclass">)  [unwired: 1 in, 1 out]
              }
              frame "PASTE" {
                # "Pastes the text from the clipboard to the active text selection"
                n96 = property class="Code String LV"(reference=w283) -> (reference out=w281:refnum<class "Code String LV.lvclass">, "Properties:Active Ref"=w282:refnum<vi>)  [unwired: 1 in, 1 out]
                n97 = call "Paste String Selection.vi"("String in"=w282) -> ("Paste Text"=w279:string)  [unwired: 12 in, 2 out]
                n98 = property class="Code String LV"(reference=w281, "Properties:Text State"=w279) -> (reference out=w280:refnum<class "Code String LV.lvclass">)  [unwired: 1 in, 1 out]
              }
            }
            n99 = call "Send Menu Selection Event.vi"("Code String in"=w248, "Item Tag"=w245, "error in (no error)"=w253) -> ("Code String out"=w247:refnum<class "Code String LV.lvclass">, "error out"=w249:errorcluster)  [unwired: 11 in]
            n100 = call <vilib>:"Add State(s) to Queue__jki_lib_state_machine.vi"("State(s) in Front (\"\")"=w246, "State(s) in (\"\")"=w251) -> ("States Out"=w252:string)  [unwired: 13 in]
          }
          event Shortcut Menu Activation? {
            # "Shortcut menu activated\nInsert user items"
            n101 = event-data() -> ("MenuRef"=w295:refnum<k9>, "CtlRef"=w291:refnum<vi>)  [unwired: 1 in]
            n102 = property class="Str"(reference=w291, error in=w289, "Key Focus"=TRUE) -> (error out=w286:errorcluster)  [unwired: 1 out]
            n103 = call "Initialize Stock Menu Items.vi"("error in (no error)"=w286, "Menu in"=w295, "Code String in"=w287) -> ("error out"=w293:errorcluster, "Menu out"=w288:refnum<k9>, "Code String out"=w285:refnum<class "Code String LV.lvclass">)  [unwired: 6 in]
            n104 = property class="Code String LV"(reference=w285) -> ("Properties:User Menu Items"=w284:T2[])  [unwired: 1 in, 2 out]
            n105 = call "Add or Remove Menu Items.vi"("error in (no error)"=w293, "Menu Items"=w284, "Menu in"=w288) -> ("error out"=w292:errorcluster)  [unwired: 7 in, 1 out]
            n106 = event-data() -> ()  [unwired: 2 in, 1 out]
          }
          event "Scrollbar": Value Change {
            # "Scrollbar value changed\nUse to set the scroll position of the other compoments"
            n107 = event-data() -> ("NewVal"=w298:i32)  [unwired: 1 in]
            n108 = Number To Decimal String(number=w298) -> (decimal integer string=w301:string)  [unwired: 1 in]
            n109 = call <vilib>:"Build State String with Arguments__jki_lib_state_machine.vi"("Arguments (\"\")"=w301, "State"="Macro: Sync Scroll") -> ("State with Arguments"=w299:string)  [unwired: 4 in]
            n110 = call <vilib>:"Add State(s) to Queue__jki_lib_state_machine.vi"("State(s) in Front (\"\")"=w299, "State(s) at Back (\"\")"="Suggestions: UI >> Cancel") -> ("States Out"=w297:string)  [unwired: 13 in]
            n111 = call <vilib>:"Add State(s) to Queue__jki_lib_state_machine.vi"("State(s) in Front (\"\")"=w297, "State(s) in (\"\")"=w305) -> ("States Out"=w306:string)  [unwired: 13 in]
          }
          event "Scrollbar": Mouse Down {
            # "Scrollbar clicked\nForce focus back to string so that we don't lose the selection"
            n112 = event-data() -> ()  [unwired: 1 in, 8 out]
            n113 = property class="Code String LV"(reference=w310) -> ("Properties:Active Ref"=w309:refnum<vi>)  [unwired: 1 in, 2 out]
            n114 = property class="Str"(reference=w309, "Key Focus"=TRUE) -> ()  [unwired: 1 in, 2 out]
          }
          event Mouse Wheel {
            # "/* At ScrollPos = 0, Delta can result in negative number.\nCoerce to 0  */"
            # "Mouse wheel scrolled\nUse to set the scroll position of the other compoments"
            n115 = event-data() -> ("Delta"=w323:i32)  [unwired: 1 in, 1 out]
            n116 = property class="Code String LV"(reference=w324) -> ("Properties:Active Ref"=w325:refnum<vi>)  [unwired: 1 in, 2 out]
            n117 = property class="Str"(reference=w325) -> ("Text.Scroll Position"=w326:u32)  [unwired: 1 in, 2 out]
            n118 = Negate(x=w323) -> (-x=w327:i32)
            n119 = To Long Integer(number=w326) -> (32bit integer=w328:i32)
            n120 = Add(x=w328, y=w327) -> (x+y=w320:i32)
            n121 = Max & Min(x=0, y=w320) -> (max(x,y)=w314:i32)  [unwired: 1 out]
            n122 = Number To Decimal String(number=w314) -> (decimal integer string=w319:string)  [unwired: 1 in]
            n123 = call <vilib>:"Build State String with Arguments__jki_lib_state_machine.vi"("Arguments (\"\")"=w319, "State"="Macro: Sync Scroll") -> ("State with Arguments"=w317:string)  [unwired: 4 in]
            n124 = call <vilib>:"Add State(s) to Queue__jki_lib_state_machine.vi"("State(s) in Front (\"\")"=w317, "State(s) at Back (\"\")"="Suggestions: UI >> Cancel") -> ("States Out"=w316:string)  [unwired: 13 in]
            n125 = call <vilib>:"Add State(s) to Queue__jki_lib_state_machine.vi"("State(s) in Front (\"\")"=w316, "State(s) in (\"\")"=w329) -> ("States Out"=w330:string)  [unwired: 13 in]
          }
          event "Line Numbers": Mouse Down? {
            # "Mouse down on line numbers\nToggle mark symbol/highlight line"
            n126 = event-data() -> ("CtlRef"=w339:refnum<vi>, "Coords"=w347:T10)  [unwired: 1 in]
            n127 = property class="LstBox (strict)"(reference=w339) -> ("Item Names"=w338:string[])  [unwired: 1 in, 2 out]
            n128 = invoke class="LstBox (strict)" method="Point To Row"(reference=w339, error in=w346, "Point"=w347) -> (reference out=w334:refnum<vi>, error out=w344:errorcluster, "Row"=w337:i32, "InGlyph"=w345:bool)  [unwired: 4 in, 3 out]
            n129 = property class="Code String LV"(reference=w333) -> ("Properties:Active Ref"=w332:refnum<vi>)  [unwired: 1 in, 2 out]
            n130 = Array Size(array=w338) -> (size(s)=w336:i32)
            n131 = Less?(x=w337, y=w336) -> (x < y?=w335:bool)
            n132 = case shown="True" w335 {
              tunnel: w332 -> [_ w354]
              tunnel: w337 -> [_ w349]
              frame False {
              }
              frame True {
                n133 = invoke class="Str" method="Get Nth Line"(reference=w354, "index"=w349) -> (reference out=w353:refnum<vi>, "start"=w351:u32, "end"=w352:u32)  [unwired: 5 in, 4 out]
                n134 = local write "Line Numbers"(w349) -> ()
                n135 = property class="Str"(reference=w353, "Key Focus"=TRUE, "Text.Selection Start"=w351, "Text.Selection End"=w352) -> ()  [unwired: 1 in, 2 out]
              }
            }
            n136 = case shown="True" w345 {
              tunnel: w337 -> [_ w360]
              tunnel: w344 -> [w355 w362]
              tunnel: w334 -> [_ w363]
              tunnel: [w355 w356] -> w343
              frame False {
              }
              frame True {
                n137 = call "Get Item Selection.vi"("error in (no error)"=w362, "Item Index"=w360, "ListBox in"=w363) -> ("error out"=w358:errorcluster, "Is Selected?"=w361:bool, "ListBox out"=w359:refnum<vi>)  [unwired: 6 in]
                n138 = Not(x=w361) -> (.not. x?=w357:bool)
                n139 = call "Set Item Selection.vi"("error in (no error)"=w358, "Is Selected?"=w357, "Item Index"=w360, "ListBox in"=w359) -> ("error out"=w356:errorcluster)  [unwired: 6 in, 1 out]
              }
            }
            n140 = event-data("Discard?"=TRUE) -> ()  [unwired: 1 in, 1 out]
            n141 = call <vilib>:"Add State(s) to Queue__jki_lib_state_machine.vi"("State(s) in (\"\")"=w340) -> ("States Out"=w341:string)  [unwired: 14 in]
          }
          event User Event {
            # "Editable setting changed\nSwitch between control/indicator visible"
            n142 = event-data() -> ()  [unwired: 1 in, 1 out]
            n143 = call <vilib>:"Add State(s) to Queue__jki_lib_state_machine.vi"("State(s) in Front (\"\")"="UI: Set Active Ref\nProcess Sync", "State(s) in (\"\")"=w366) -> ("States Out"=w367:string)  [unwired: 13 in]
          }
          event User Event {
            # "Font size changed\nUpdate the font size of the existing text, resize  the UI to have complete lines, update the scrollbar range/value"
            n144 = event-data() -> ()  [unwired: 1 in, 1 out]
            n145 = call <vilib>:"Add State(s) to Queue__jki_lib_state_machine.vi"("State(s) in Front (\"\")"="UI: Set Font Size\nUI: Resize\nUI: Adjust Line Numbers\nMacro: Navigate Lines\nSuggestions: UI >> Font", "State(s) in (\"\")"=w371) -> ("States Out"=w372:string)  [unwired: 13 in]
          }
          event User Event {
            # "Font color changed\nUpdate the font color of the current text selection"
            n146 = event-data() -> ("Font Color"=w378:u32)  [unwired: 1 in]
            n147 = Number To Decimal String(number=w378) -> (decimal integer string=w377:string)  [unwired: 1 in]
            n148 = call <vilib>:"Build State String with Arguments__jki_lib_state_machine.vi"("Arguments (\"\")"=w377, "State"="UI: Set Font Color") -> ("State with Arguments"=w376:string)  [unwired: 4 in]
            n149 = call <vilib>:"Add State(s) to Queue__jki_lib_state_machine.vi"("State(s) in Front (\"\")"=w376, "State(s) in (\"\")"=w380) -> ("States Out"=w381:string)  [unwired: 13 in]
          }
          event User Event {
            # "Text selection start changed\nUpdate the selection"
            n150 = event-data() -> ("Selection Start"=w390:u32)  [unwired: 1 in]
            n151 = Format Into String(format string="Start = %d", w390) -> (resulting string=w388:string)  [unwired: 2 in, 1 out]
            n152 = call <vilib>:"Build State String with Arguments__jki_lib_state_machine.vi"("Arguments (\"\")"=w388, "State"="UI: Set Selection") -> ("State with Arguments"=w386:string)  [unwired: 4 in]
            n153 = call <vilib>:"Add State(s) to Queue__jki_lib_state_machine.vi"("State(s) in (\"\")"=w386, "State(s) at Back (\"\")"="Process Sync" ("State(s) at Back (\"\")")) -> ("States Out"=w387:string)  [unwired: 13 in]
            n154 = call <vilib>:"Add State(s) to Queue__jki_lib_state_machine.vi"("State(s) in Front (\"\")"=w387, "State(s) in (\"\")"=w392) -> ("States Out"=w393:string)  [unwired: 13 in]
          }
          event User Event {
            # "Text selection end changed\nUpdate the selection"
            n155 = event-data() -> ("Selection End"=w402:u32)  [unwired: 1 in]
            n156 = Format Into String(format string="End = %d", w402) -> (resulting string=w400:string)  [unwired: 2 in, 1 out]
            n157 = call <vilib>:"Build State String with Arguments__jki_lib_state_machine.vi"("Arguments (\"\")"=w400, "State"="UI: Set Selection") -> ("State with Arguments"=w398:string)  [unwired: 4 in]
            n158 = call <vilib>:"Add State(s) to Queue__jki_lib_state_machine.vi"("State(s) in (\"\")"=w398, "State(s) at Back (\"\")"="Process Sync" ("State(s) at Back (\"\")")) -> ("States Out"=w399:string)  [unwired: 13 in]
            n159 = call <vilib>:"Add State(s) to Queue__jki_lib_state_machine.vi"("State(s) in Front (\"\")"=w399, "State(s) in (\"\")"=w404) -> ("States Out"=w405:string)  [unwired: 13 in]
          }
          event User Event {
            # "Scrollbar value changed programmatically\nUse to set the scroll position of the other compoments"
            n160 = event-data() -> ("Scroll Position"=w410:u32)  [unwired: 1 in]
            n161 = Number To Decimal String(number=w410) -> (decimal integer string=w413:string)  [unwired: 1 in]
            n162 = call <vilib>:"Build State String with Arguments__jki_lib_state_machine.vi"("Arguments (\"\")"=w413, "State"="Macro: Sync Scroll") -> ("State with Arguments"=w411:string)  [unwired: 4 in]
            n163 = call <vilib>:"Add State(s) to Queue__jki_lib_state_machine.vi"("State(s) in Front (\"\")"=w411, "State(s) at Back (\"\")"="Suggestions: UI >> Cancel") -> ("States Out"=w409:string)  [unwired: 13 in]
            n164 = call <vilib>:"Add State(s) to Queue__jki_lib_state_machine.vi"("State(s) in Front (\"\")"=w409, "State(s) in (\"\")"=w416) -> ("States Out"=w417:string)  [unwired: 13 in]
          }
          event User Event {
            # "String received\nReplace text and process"
            n165 = event-data() -> ()  [unwired: 1 in, 1 out]
            n166 = call <vilib>:"Add State(s) to Queue__jki_lib_state_machine.vi"("State(s) in Front (\"\")"="Macro: Process Text >> Move Cursor\nProcess Sync", "State(s) in (\"\")"=w422) -> ("States Out"=w423:string)  [unwired: 13 in]
          }
          event User Event {
            # "String received\nReplace text and process"
            n167 = event-data() -> ()  [unwired: 1 in, 1 out]
            n168 = call <vilib>:"Add State(s) to Queue__jki_lib_state_machine.vi"("State(s) in Front (\"\")"="UI: Insert String\nMacro: Process Text\nProcess Sync", "State(s) in (\"\")"=w428) -> ("States Out"=w429:string)  [unwired: 13 in]
          }
          event User Event {
            # "Menu items received\nAdd to the User Menu Items lookup"
            n169 = event-data() -> ("Item Path"=w437:string, "Visible?"=w435:bool, "Checked?"=w436:bool)  [unwired: 1 in]
            n170 = Bundle By Name(cluster=T2 {"Item Path"="", "Visible?"=FALSE, "Checked?"=FALSE} ("Menu Item"), "Item Path"=w437, "Visible?"=w435, "Checked?"=w436) -> (w433:T2)
            n171 = Build Array(w433) -> (w432:T2[])
            n172 = property class="Code String LV"(reference=w441, "Properties:User Menu Items"=w432) -> (reference out=w439:refnum<class "Code String LV.lvclass">)  [unwired: 1 in, 1 out]
          }
          event User Event {
            # "Selection sent from suggestion panel\nInsert into the main string"
            n173 = event-data() -> ("Suggestion"=w445:string)  [unwired: 1 in]
            n174 = Empty String/Path?(string/path=w445) -> (empty?=w444:bool)
            n175 = Bundle By Name(cluster=w452, "Suggestions.Visible?"=FALSE, "Suggestions.Selected"=w445) -> (w449:T14)
            n176 = case shown="False" w444 {
              tunnel: ["UI: Insert String >> Suggestion\nMacro: Process Text" _] -> w446
              frame False {
              }
              frame True {
              }
            }
            n177 = call <vilib>:"Add State(s) to Queue__jki_lib_state_machine.vi"("State(s) in Front (\"\")"=w446, "State(s) in (\"\")"=w447) -> ("States Out"=w448:string)  [unwired: 13 in]
          }
          event User Event {
            # "Stop the panel\nSync if requested"
            n178 = event-data() -> ("Sync on Exit?"=w460:bool)  [unwired: 1 in]
            n179 = Select(t="Sync", s=w460, f="") -> (s? t:f=w457:string)
            n180 = call <vilib>:"Build State String with Arguments__jki_lib_state_machine.vi"("Arguments (\"\")"=w457, "State"="Macro: Exit") -> ("State with Arguments"=w455:string)  [unwired: 4 in]
            n181 = call <vilib>:"Add State(s) to Queue__jki_lib_state_machine.vi"("State(s) in Front (\"\")"=w455, "State(s) in (\"\")"=w461) -> ("States Out"=w462:string)  [unwired: 13 in]
          }
          event Panel Close? {
            # "Close Panel button (pressed) Event\n(this executes Macro: Exit to terminate the VI)"
            n182 = event-data() -> ()  [unwired: 1 in, 1 out]
            n183 = event-data("Discard?"=TRUE) -> ()  [unwired: 1 in, 1 out]
            n184 = call <vilib>:"Add State(s) to Queue__jki_lib_state_machine.vi"("State(s) in Front (\"\")"="Macro: Exit", "State(s) in (\"\")"=w471) -> ("States Out"=w470:string)  [unwired: 13 in]
          }
        }
      }
      frame "---------- Core ----------" {
        # "Do not put any code in this frame.\n(it is a separator no-op)"
        n185 = call <vilib>:"Add State(s) to Queue__jki_lib_state_machine.vi"("State(s) in (\"\")"=w477) -> ("States Out"=w476:string)  [unwired: 14 in]
      }
      frame Default {
        w489 = 42 items=["No error", "Argument error", "Memory is full", "Out of zone", "End of file", "File already open", "Generic file I/O error", "File not found", "File permission error", "Disk is full", "Duplicate path", "Too many files open", "System feature not enabled", "Resource file not found", "Cannot add resource", "Resource not found", "Image not found", "Image memory error", "Pen does not exist", "Config type invalid", "Config token not found", "Config parse error", "Config memory error", "Bad external code format", "Bad external code offset", "External code not present", "Null window", "Destroy window error", "Null menu", "Print aborted", "Bad print record", "Print driver error", "Windows error during printing", "Memory error during printing", "Print dialog error", "Generic print error", "Invalid device refnum", "Device not found", "Device parameter error", "Device unit error", "Cannot open device", "Device call aborted", "Generic error", "Cancelled by user", "Object ID too low", "Object ID too high", "Object not in heap", "Unknown heap", "Unknown object (invalid DefProc)", "Unknown object (DefProc not in table)", "Message out of range", "Invalid (null) method", "Unknown message", "Manager call not supported", "Bad address", "Network operation in progress", "Network operation timed out", "Connection is busy", "Network attribute not supported", "Network error", "Address in use", "System out of memory", "Connection aborted", "Connection refused", "Not connected", "Already connected", "Connection closed", "Initialization error (interapplication manager)", "Bad occurrence", "Wait on unbound occurrence handler", "Occurrence queue overflow", "Datalog type conflict", "Unused", "Unrecognized type (interapplication manager)", "Memory corrupt", "Failed to make temporary DLL", "Old CIN version", "Drag socket not found", "Failed to load drop-object", "Failed to register OLE object", "Failed to release OLE object", "Format specifier type mismatch", "Unknown format specifier", "Too few format specifiers", "Too many format specifiers", "Scan failed", "Newer CIN version", "Error converting to variant", "Runtime menu error", "Password tampered", "Variant attribute not found", "Incompatible variant data type", "Event data is not available", "Event Store is not present", "Occurrence is not found", "Event Queue is not created", "Event info is not available", "Refnum passed is NULL", "Error retrieving Class GUID", "Error retrieving CoClass GUID", "Error retrieving TypeLib GUID.", "Bad built application magic bytes.", "Specific driver is different from the specific driver associated with the Logical Name.", "There is no session opened to the class driver.", "Max Error", "MAX - Error with config objects", "MAX - Error loading configuration", "MAX - Group not supported"]
        # "Current State"
        # "Do not delete, rename, or modify this frame.\n(this is used to capture unhandled states and typos)"
        # "Handle mistyped state name (developer tool)"
        n186 = Format Into String(format string="Software Exception: Unhandled State \"%s\"." ("message"), error in=w485, w480) -> (resulting string=w488:string, error out=w487:errorcluster)  [unwired: 1 in]
        n187 = call <vilib>:"Error Cluster From Error Code.vi"("show call chain? (False)"=TRUE, "error in (no error)"=w487, "error message (\"\")"=w488, "error code (0)"=w489) -> ("error out"=w486:errorcluster)  [unwired: 5 in]
        n188 = call <vilib>:"Add State(s) to Queue__jki_lib_state_machine.vi"("State(s) in (\"\")"=w484) -> ("States Out"=w483:string)  [unwired: 14 in]
      }
      frame "Initialize Core Data" {
        # "Do not delete, rename, or modify this frame.\n(this is used to determine panel behavior on exit)"
        # "originally closed?"
        # "exe?"
        # "If panel starts closed or is an EXE, then close it when we exit"
        n189 = property class="VI"() -> ("FP.State"=w495:T3)  [unwired: 2 in, 2 out]
        n190 = property class="App"() -> ("App.Kind"=w501:T4)  [unwired: 2 in, 2 out]
        n191 = control-ref of="Current VI Reference"() -> (w496:refnum<vi>)
        n192 = Equal?(x=w495, y=T3."Closed" ("Front Panel Window:State")) -> (x = y?=w493:bool)
        n193 = Equal?(x=w501, y=T4."Run Time System" ("Application:Kind")) -> (x = y?=w499:bool)
        n194 = Or(x=w493, y=w499) -> (x .or. y?=w497:bool)
        n195 = Bundle By Name(cluster=w498, "Core.Current VI Reference"=w496, "Core.Close Panel on Exit?"=w497) -> (w503:T14)
        n196 = call <vilib>:"Add State(s) to Queue__jki_lib_state_machine.vi"("State(s) in (\"\")"=w505) -> ("States Out"=w504:string)  [unwired: 14 in]
      }
      frame "Process Sync" {
        # "Wait on rendezvous\nCalled to synchronize with external process"
        n197 = property class="Code String LV"(reference=w507) -> ("Properties:Rendezvous"=w506:T16)  [unwired: 1 in, 2 out]
        n198 = call <vilib>:"Wait at Rendezvous.vi"("error in (no error)"=w509, "ms timeout (-1)"=500, "rendezvous"=w506) -> ("error out"=w508:errorcluster)  [unwired: 2 in, 2 out]
        n199 = call <vilib>:"Add State(s) to Queue__jki_lib_state_machine.vi"("State(s) in (\"\")"=w514) -> ("States Out"=w513:string)  [unwired: 14 in]
      }
      frame "Error Handler" {
        # "Unhandled Error -- Display it"
        # "Handle any errors here.\nYou can also output any states to clean-up after errors occur"
        # "Clear error"
        n200 = call <vilib>:"General Error Handler.vi"("error in (no error)"=w518) -> ()  [unwired: 10 in, 5 out]
        n201 = call <vilib>:"Add State(s) to Queue__jki_lib_state_machine.vi"("State(s) in Front (\"\")"="/* Post Error States", "State(s) in (\"\")"=w522) -> ("States Out"=w521:string)  [unwired: 13 in]
      }
      frame "Exit" {
        # "Do not put any code in this frame.\n(No errors that occur here will be handled.)"
        n202 = call <vilib>:"Add State(s) to Queue__jki_lib_state_machine.vi"("State(s) in (\"\")"=w529) -> ("States Out"=w528:string)  [unwired: 14 in]
      }
      frame "---------- Data ----------" {
        # "Do not put any code in this frame.\n(It is a separator no-op. You can make a copy of this frame to create a new Data frame)"
        n203 = call <vilib>:"Add State(s) to Queue__jki_lib_state_machine.vi"("State(s) in (\"\")"=w535) -> ("States Out"=w534:string)  [unwired: 14 in]
      }
      frame "Data: Initialize" {
        w536 = cluster{"?":bool, "Offset":T6, "Bounds":T13} {"?"=FALSE, "Offset"={"Horizontal"=0, "Vertical"=0}, "Bounds"={"Left"=0, "Top"=0, "Right"=0, "Bottom"=0}}  # Mouse Down
        w541 = refnum<vi>[] []  # Strings
        w544 = -1  # T
        w547 = refnum<vi>[] []  # Panes
        w537 = T17 {"Suggestion Box"=refnum, "Visible?"=FALSE, "Display Limit"=0, "Update Data"={"Query"="", "Keywords"=[], "Position"={"Left"=0, "Top"=0}}, "Selected"="", "Location"={"Selection Start"=0, "Selection End"=0}, "Delta?"=FALSE}  # Suggestions
        w554 = T18 {"Current VI Reference"=refnum, "Close Panel on Exit?"=FALSE}  # Core
        # "Initialize the shift-register data, here.\n(data names are defined by what you wire into the bundle function)"
        n204 = control-ref of="Scrollbar"() -> (w538:refnum<vi>)
        n205 = control-ref of="Line #"() -> (w539:refnum<vi>)
        n206 = control-ref of="String Indicator"() -> (w546:refnum<vi>)
        n207 = control-ref of="String Control"() -> (w545:refnum<vi>)
        n208 = control-ref of="Line Pane"() -> (w551:refnum<vi>)
        n209 = control-ref of="Text Pane"() -> (w550:refnum<vi>)
        n210 = control-ref of="Scroll Pane"() -> ()  [unwired: 1 out]
        n211 = Build Array(w551, w550) -> (w549:refnum<vi>[])
        n212 = Build Array(w546, w545) -> (w542:refnum<vi>[])
        n213 = Type Cast(type=w547, x=w549) -> (*(type *) &x=w548:refnum<vi>[])
        n214 = Type Cast(type=w541, x=w542) -> (*(type *) &x=w540:refnum<vi>[])
        n215 = Bundle("Core"=w554, "T"=w544, "Panes"=w548, "Strings"=w540, "Line #"=w539, "Scrollbar"=w538, "Suggestions"=w537, "Mouse Down"=w536) -> (w556:T14)  [unwired: 1 in]
        "String Indicator" <- "String Control"
      }
      frame "Data: Register Events" {
        # "Register for dynamic events\nUser events and UI events"
        n216 = Unbundle By Name(w567) -> ("Strings"=w561:refnum<vi>[], "Panes"=w559:refnum<vi>[], "Suggestions.Suggestion Box"=w566:refnum<class "Suggestion Box.lvclass">)
        n217 = property class="Code String LV"(reference=w558) -> ("Properties:User Events"=w560:T19)  [unwired: 1 in, 2 out]
        n218 = call "Read Public Events.vi"("error in (no error)"=w563, "Suggestion Box in"=w566) -> ("error out"=w564:errorcluster, "Public Events"=w565:T20)  [unwired: 7 in, 1 out]
        n219 = register-events(error in=w564, w560, w561, w561, w561, w561, w561, w561, w561, w561, w561, w559, w559, w565) -> (reference out=w562:refnum<event-registration>, error out=w568:errorcluster)  [unwired: 1 in]
        n220 = call <vilib>:"Add State(s) to Queue__jki_lib_state_machine.vi"("State(s) in (\"\")"=w570) -> ("States Out"=w569:string)  [unwired: 14 in]
      }
      frame "Data: Update Selection" {
        # "Updates the selected lines/token\nCan be with respect to the text selection indices (character offsets) or on-screen coordinates"
        n221 = property class="Code String LV"(reference=w586) -> (reference out=w585:refnum<class "Code String LV.lvclass">, "Properties:Active Ref"=w577:refnum<vi>, "Properties:Delimiter Pattern"=w584:string)  [unwired: 1 in, 1 out]
        n222 = case shown="\"\"" w582 {
          selector: w582 -> [_ w614]
          tunnel: w584 -> [w604 w607]
          tunnel: w577 -> [w603 w608]
          tunnel: [w602 w605] -> w574
          tunnel: [w601 w606] -> w583
          tunnel: [w600 w615] -> w578
          tunnel: [w599 w609] -> w576
          frame "" {
            # "/* No coordinates supplied, use the string's text selection indices */"
            n223 = call "Get Lines from Selection.vi"("String in"=w603, "Delimiter Regular Expression"=w604) -> ("Selected Lines"=w602:string, "# Lines"=w601:i32, "Selected Token"=w600:string, "Selected Text"=w599:string)  [unwired: 9 in, 1 out]
          }
          frame Default {
            n224 = Scan From String(format string="(%d, %d)", input string=w614) -> (output 1=w612:i32, output 2=w611:i32)  [unwired: 4 in, 3 out]
            n225 = Bundle(w612, w611) -> (w610:cluster{i32, i32})  [unwired: 1 in]
            n226 = call "Get Lines from Selection.vi"("String in"=w608, "Delimiter Regular Expression"=w607) -> ("Selected Lines"=w605:string, "# Lines"=w606:i32, "Selected Text"=w609:string)  [unwired: 9 in, 2 out]
            n227 = call "Get Lines from Point.vi"("String in"=w608, "Delimiter Regular Expression"=w607, "Point"=w610) -> ("Selected Token"=w615:string)  [unwired: 8 in, 4 out]
          }
        }
        n228 = call-poly <userlib>:"Data Changed__ogtk.vi"("String"=w574) -> ("Changed"=w573:bool)
        n229 = property class="Code String LV"(reference=w585, "Properties:Selected Line(s)"=w574, "Properties:# Selected Lines"=w583, "Properties:Selected Token"=w578, "Properties:Selected Text State"=w576) -> (reference out=w580:refnum<class "Code String LV.lvclass">)  [unwired: 1 in, 1 out]
        n230 = Bundle By Name(cluster=w588, "Suggestions.Delta?"=w573) -> (w575:T14)
        n231 = call "Enough Time Passed.vi"("Timeout"=u32 200 ("y")) -> ("Timed out?"=w571:bool)
        n232 = case shown="False" w571 {
          tunnel: w589 -> [w592 w598]
          tunnel: [w592 w597] -> w581
          tunnel: w580 -> [w593 w596]
          tunnel: [w593 w595] -> w579
          tunnel: w578 -> [_ w594]
          frame False {
          }
          frame True {
            n233 = call "Send Selected Token Changed Event.vi"("Code String in"=w596, "Selected Token"=w594, "error in (no error)"=w598) -> ("Code String out"=w595:refnum<class "Code String LV.lvclass">, "error out"=w597:errorcluster)  [unwired: 11 in]
          }
        }
        n234 = call <vilib>:"Add State(s) to Queue__jki_lib_state_machine.vi"("State(s) in (\"\")"=w591) -> ("States Out"=w590:string)  [unwired: 14 in]
      }
      frame "Data: Set String State" {
        # "When typing, the following event sequence occurs:\n- <Strings> Key Down?\n- <Strings> Key Down\n- <Strings> Value Change\nWe want 'Key Down' and 'Value Change' to do the same thing to handle Copy/Paste,\nso we can flush the Value Change when Key Down has just occurred."
        # "Pass the active string value to the state data (DVR)\nFlush value change events to avoid duplicate processing for key down/value change"
        n235 = property class="Code String LV"(reference=w622) -> (reference out=w623:refnum<class "Code String LV.lvclass">, "Properties:Active Ref"=w624:refnum<vi>)  [unwired: 1 in, 1 out]
        n236 = property class="Str"(reference=w624) -> ("Value"=w616:string)  [unwired: 1 in, 2 out]
        n237 = property class="Code String LV"(reference=w623, "Properties:Text State"=w616) -> (reference out=w621:refnum<class "Code String LV.lvclass">)  [unwired: 1 in, 1 out]
        n238 = disable-structure shown="Enabled" {
          disable-tunnel: w620 -> [w632 w633]
          disable-tunnel: [w631 w633] -> w619
          disable-tunnel: w618 -> [w629 _]
          disable-tunnel: [w628 _] -> w617
          frame Enabled {
            n239 = Flush Event Queue(0:w632, 2:lveventtype."Value Change" ("event type or object"), 3:w629) -> (8:w631:refnum<event-registration>, 11:w628:errorcluster)  [unwired: 3 in, 1 out]
          }
          frame Disabled {
          }
        }
        n240 = call <vilib>:"Add State(s) to Queue__jki_lib_state_machine.vi"("State(s) in (\"\")"=w627) -> ("States Out"=w626:string)  [unwired: 14 in]
      }
      frame "Data: Cleanup" {
        # "Cleanup any data and references, here.\n(this is called automatically, by the Macro: Exit)"
        n241 = Unregister For Events(event registration refnum=w634, error in=w639) -> (error out=w635:errorcluster)
        n242 = Unbundle By Name(w637) -> ("Core.Current VI Reference"=w640:refnum<vi>)
        n243 = Close Reference(reference=w640, error in (no error)=w635) -> (error out=w638:errorcluster)
        n244 = call <vilib>:"Add State(s) to Queue__jki_lib_state_machine.vi"("State(s) in (\"\")"=w642) -> ("States Out"=w641:string)  [unwired: 14 in]
      }
      frame "---------- UI ----------" {
        # "Do not put any code in this frame.\n(It is a separator no-op. You can make a copy of this frame to create a new UI frame)"
        n245 = call <vilib>:"Add State(s) to Queue__jki_lib_state_machine.vi"("State(s) in (\"\")"=w648) -> ("States Out"=w647:string)  [unwired: 14 in]
      }
      frame "UI: Initialize" {
        w657 = 0.0 ("Doc Min")
        w665 = TRUE ("Coerce Minimum Value")
        # "Initialize the User Interface, here.\n(this is called automatically, by the Macro: Init)"
        n246 = Unbundle By Name(w650) -> ("Strings"=w655:refnum<vi>[], "Line #"=w667:refnum<vi>, "Scrollbar"=w661:refnum<vi>)
        n247 = global read "Font Global.vi" "Font Size"() -> (w652:u32)
        n248 = call "Populate Line Numbers.vi"("Line Numbers in"=w667, "Total Number of Lines"=0) -> ("Line Numbers out"=w663:refnum<vi>)  [unwired: 13 in]
        n249 = global read "Font Global.vi" "Font"() -> (w651:string)
        n250 = Decrement(x=w652) -> (x-1=w653:u32)
        n251 = for {
          tunnel: w655 -> [w684] mode=indexing
          tunnel: "" -> [w683]
          tunnel: w651 -> [w682]
          tunnel: w652 -> [w681]
          tunnel: u32 0 -> [w680]
          n252 = property class="Str"(reference=w684, "Value"=w683, "Text.FontName"=w682, "Text.FontSize"=w681, "Text.FontColor"=w680) -> ()  [unwired: 1 in, 2 out]
        }
        n253 = property class="LstBox (strict)"(reference=w663, "Value"=0, "Active Row"=-2 ("Active Row:Active Row Number"), "Cell Height"=w653, "CellFontName"=w651, "CellFontSize"=w652, "Justify"=enum16{"Left", "Center", "Right"}."Right" ("Active Row:Cell Justification")) -> (reference out=w662:refnum<vi>)  [unwired: 1 in, 1 out]
        n254 = property class="Scroll (strict)"(reference=w661, "PageSize"=10.0 ("Doc Min"), "Increment"=1.0, "DocMax"=w657, "DocMin"=w657, "CoerceMin"=w665, "CoerceMax"=w665, "Value"=0) -> ()  [unwired: 1 in, 2 out]
        n255 = call "Populate Line Numbers.vi"("Line Numbers in"=w662, "Total Number of Lines"=1 ("dimension size")) -> ()  [unwired: 13 in, 1 out]
        n256 = disable-structure shown="Enabled" {
          frame Disabled {
            n257 = control-ref of="This VI"() -> (w677:refnum<vi>)
            n258 = property class="VI"(reference=w677) -> ("Panel"=w676:refnum<vi>)  [unwired: 1 in, 2 out]
            n259 = property class="Pnl"(reference=w676) -> ("Panes[]"=w675:refnum<vi>[])  [unwired: 1 in, 2 out]
            n260 = for {
              tunnel: w675 -> [w679] mode=indexing
              n261 = property class="Pane"(reference=w679, "Origin"=T6 {"Horizontal"=0, "Vertical"=0}) -> ()  [unwired: 1 in, 2 out]
            }
          }
          frame Enabled {
          }
        }
        n262 = call <vilib>:"Add State(s) to Queue__jki_lib_state_machine.vi"("State(s) in (\"\")"=w674) -> ("States Out"=w673:string)  [unwired: 14 in]
      }
      frame "UI: Cursor Set" {
        # "Argument"
        # "Set and Unset Cursor Busy.\n(Usage: \"UI: Cursor Set >> Busy|Idle\")"
        n263 = case shown="\"Idle\", Default" w687 {
          tunnel: w689 -> [w694 w696]
          tunnel: [w693 w695] -> w688
          frame "Idle", Default {
            n264 = call <vilib>:"Unset Busy.vi"("error in (no error)"=w694) -> ("error out"=w693:errorcluster)  [unwired: 10 in]
          }
          frame "Busy" {
            n265 = call <vilib>:"Set Busy.vi"("error in (no error)"=w696) -> ("error out"=w695:errorcluster)  [unwired: 9 in, 1 out]
          }
        }
        n266 = call <vilib>:"Add State(s) to Queue__jki_lib_state_machine.vi"("State(s) in (\"\")"=w692) -> ("States Out"=w691:string)  [unwired: 14 in]
      }
      frame "UI: Front Panel State" {
        # "Argument"
        # "Set Front Panel Open or Closed\n(Usage: \"UI: Front Panel State >> Open|Close\")"
        n267 = Unbundle By Name(w701) -> ("Core.Current VI Reference"=w700:refnum<vi>)
        n268 = case shown="\"Close\", \"Closed\"" w699 {
          tunnel: w703 -> [w711 w726 w737 w750 w763]
          tunnel: [w713 w727 w739 w752 w765] -> w702
          tunnel: w700 -> [w712 w724 w738 w751 w764]
          frame "Open", "Standard", Default {
            w706 = T3."Standard" ("State")
            n269 = property class="VI"(reference=w712, error in=w711) -> (reference out=w709:refnum<vi>, error out=w710:errorcluster, "FP.State"=w708:T3)
            n270 = Not Equal?(x=w708, y=w706) -> (x != y?=w707:bool)
            n271 = case shown="True" w707 {
              tunnel: [w717 w719] -> w713
              tunnel: w710 -> [w716 w719]
              tunnel: w709 -> [w715 _]
              tunnel: w706 -> [w714 _]
              frame True {
                n272 = invoke class="VI" method="FP.Open"(reference=w715, error in=w716, "Activate"=TRUE, "State"=w714) -> (error out=w717:errorcluster)  [unwired: 1 in, 4 out]
              }
              frame False {
              }
            }
          }
          frame "Close", "Closed" {
            n273 = property class="VI"(reference=w724, error in=w726) -> (reference out=w723:refnum<vi>, error out=w725:errorcluster, "FP.State"=w721:T3)
            n274 = Not Equal?(x=w721, y=T3."Closed" ("Front Panel Window:State")) -> (x != y?=w720:bool)
            n275 = case shown="True" w720 {
              tunnel: [w728 w731] -> w727
              tunnel: w725 -> [w728 w730]
              tunnel: w723 -> [_ w729]
              frame False {
              }
              frame True {
                n276 = invoke class="VI" method="FP.Close"(reference=w729, error in=w730) -> (error out=w731:errorcluster)  [unwired: 1 in, 2 out]
              }
            }
          }
          frame "Hidden", "Hide" {
            w732 = T3."Hidden" ("State")
            n277 = property class="VI"(reference=w738, error in=w737) -> (reference out=w735:refnum<vi>, error out=w736:errorcluster, "FP.State"=w734:T3)
            n278 = Not Equal?(x=w734, y=w732) -> (x != y?=w733:bool)
            n279 = case shown="True" w733 {
              tunnel: [w743 w744] -> w739
              tunnel: w736 -> [w742 w744]
              tunnel: w735 -> [w741 _]
              tunnel: w732 -> [w740 _]
              frame True {
                n280 = invoke class="VI" method="FP.Open"(reference=w741, error in=w742, "State"=w740) -> (error out=w743:errorcluster)  [unwired: 2 in, 4 out]
              }
              frame False {
              }
            }
          }
          frame "Minimize", "Minimized" {
            w745 = T3."Minimized" ("State")
            n281 = property class="VI"(reference=w751, error in=w750) -> (reference out=w748:refnum<vi>, error out=w749:errorcluster, "FP.State"=w747:T3)
            n282 = Not Equal?(x=w747, y=w745) -> (x != y?=w746:bool)
            n283 = case shown="True" w746 {
              tunnel: [w756 w757] -> w752
              tunnel: w749 -> [w755 w757]
              tunnel: w748 -> [w754 _]
              tunnel: w745 -> [w753 _]
              frame True {
                n284 = invoke class="VI" method="FP.Open"(reference=w754, error in=w755, "State"=w753) -> (error out=w756:errorcluster)  [unwired: 2 in, 4 out]
              }
              frame False {
              }
            }
          }
          frame "Maximize", "Maximized" {
            w758 = T3."Maximized" ("State")
            n285 = property class="VI"(reference=w764, error in=w763) -> (reference out=w761:refnum<vi>, error out=w762:errorcluster, "FP.State"=w760:T3)
            n286 = Not Equal?(x=w760, y=w758) -> (x != y?=w759:bool)
            n287 = case shown="True" w759 {
              tunnel: [w769 w770] -> w765
              tunnel: w762 -> [w768 w770]
              tunnel: w761 -> [w767 _]
              tunnel: w758 -> [w766 _]
              frame True {
                n288 = invoke class="VI" method="FP.Open"(reference=w767, error in=w768, "State"=w766) -> (error out=w769:errorcluster)  [unwired: 2 in, 4 out]
              }
              frame False {
              }
            }
          }
        }
        n289 = call <vilib>:"Add State(s) to Queue__jki_lib_state_machine.vi"("State(s) in (\"\")"=w705) -> ("States Out"=w704:string)  [unwired: 14 in]
      }
      frame "UI: Defer Updates" {
        # "Defer panel updates\n(Usage: \"UI: Defer Updates >> True|False\")"
        n290 = Unbundle By Name(w779) -> ("Core.Current VI Reference"=w772:refnum<vi>)
        n291 = case shown="\"True\"" w780 {
          tunnel: [FALSE TRUE] -> w773
          frame "False", Default {
          }
          frame "True" {
          }
        }
        n292 = property class="VI"(reference=w772, error in=w774) -> (error out=w777:errorcluster, "Panel"=w778:refnum<vi>)  [unwired: 1 out]
        n293 = property class="Pnl"(reference=w778, error in=w777, "DeferPanUpdts"=w773) -> (reference out=w775:refnum<vi>, error out=w776:errorcluster)
        n294 = Close Reference(reference=w775, error in (no error)=w776) -> (error out=w771:errorcluster)
        n295 = call <vilib>:"Add State(s) to Queue__jki_lib_state_machine.vi"("State(s) in (\"\")"=w784) -> ("States Out"=w783:string)  [unwired: 14 in]
      }
      frame "UI: Set Active Ref" {
        w793 = TRUE
        # "#note Control is index 1, Indicator is index 0"
        # "/* Update visibility from back to front to avoid flicker */"
        # "Set the indicator or control to be the active component\nCalled when changing the Editable property"
        n296 = property class="Code String LV"(reference=w788) -> ("Properties:Editable"=w790:bool)  [unwired: 1 in, 2 out]
        n297 = Unbundle By Name(w787) -> ("Strings"=w797:refnum<vi>[])
        n298 = Index Array(array=w797) -> (element #1=w795:refnum<vi>, element #2=w796:refnum<vi>)  [unwired: 2 in]
        n299 = Swap Values(12:w795, 13:w790, 14:w796) -> (1:w789:refnum<vi>, 3:w791:refnum<vi>)
        n300 = property class="Str"(reference=w789, "Visible"=w793) -> (error out=w794:errorcluster)  [unwired: 1 in, 1 out]
        n301 = property class="Code String LV"(reference=w788, "Properties:Active Ref"=w789) -> ()  [unwired: 1 in, 2 out]
        n302 = Not(x=w793) -> (.not. x?=w792:bool)
        n303 = property class="Str"(reference=w791, error in=w794, "Visible"=w792) -> ()  [unwired: 2 out]
        n304 = call <vilib>:"Add State(s) to Queue__jki_lib_state_machine.vi"("State(s) in (\"\")"=w801) -> ("States Out"=w800:string)  [unwired: 14 in]
      }
      frame "UI: Resize" {
        # "Size the UI components to fit nicely\nCall during initialization and when the pane is resized"
        n305 = Unbundle By Name(w815) -> ("Core.Current VI Reference"=w804:refnum<vi>, "Line #"=w807:refnum<vi>, "Scrollbar"=w808:refnum<vi>, "Strings"=w809:refnum<vi>[])
        n306 = control-ref of="Decoration"() -> (w806:refnum<vi>)
        n307 = disable-structure shown="Enabled" {
          disable-tunnel: w811 -> [w823 w824]
          disable-tunnel: w809 -> [w822 _]
          disable-tunnel: w808 -> [w821 _]
          disable-tunnel: w807 -> [w820 _]
          disable-tunnel: w806 -> [w819 _]
          disable-tunnel: [w818 w824] -> w805
          disable-tunnel: w804 -> [w817 _]
          frame Enabled {
            n308 = call "Size UI.vi"("VI"=w817, "Decoration"=w819, "Line Numbers"=w820, "Scrollbar"=w821, "Strings"=w822, "error in (no error)"=w823) -> ("error out"=w818:errorcluster)  [unwired: 9 in]
          }
          frame Disabled {
          }
        }
        n309 = Flush Event Queue(0:w813, 2:lveventtype."Pane Size" ("event type or object"), 3:w805, 5:1 ("keep most recent")) -> (8:w812:refnum<event-registration>, 11:w810:errorcluster)  [unwired: 2 in, 1 out]
      }
      frame "UI: Insert String" {
        # "Insert selected suggestion into string\nCall after accepting a suggestion. Location provided by Suggestions:Search"
        n310 = case shown="Default" w826 {
          tunnel: w834 -> [_ w847]
          tunnel: [w839 w846] -> w833
          tunnel: [w841 w845] -> w832
          tunnel: w828 -> [w843 w844]
          tunnel: [w842 w844] -> w827
          frame Default {
            n311 = property class="Code String LV"(reference=w843) -> (reference out=w842:refnum<class "Code String LV.lvclass">, "Properties:Selected Text"=w841:string, "Properties:Active Ref"=w840:refnum<vi>)  [unwired: 1 in, 1 out]
            n312 = property class="Str"(reference=w840) -> ("Text.Selection"=w839:T12)  [unwired: 1 in, 2 out]
          }
          frame "Suggestion" {
            n313 = Unbundle By Name(w847) -> ("Suggestions.Selected"=w845:string, "Suggestions.Location"=w846:T12)
          }
        }
        n314 = property class="Code String LV"(reference=w827) -> (reference out=w830:refnum<class "Code String LV.lvclass">, "Properties:Active Ref"=w831:refnum<vi>)  [unwired: 1 in, 1 out]
        n315 = call "Change String.vi"("String in"=w831, "Insertion"=w832, "Location"=w833) -> ("Result"=w825:string)  [unwired: 11 in, 1 out]
        n316 = property class="Code String LV"(reference=w830, "Properties:Text State"=w825) -> (reference out=w829:refnum<class "Code String LV.lvclass">)  [unwired: 1 in, 1 out]
        n317 = call <vilib>:"Add State(s) to Queue__jki_lib_state_machine.vi"("State(s) in (\"\")"=w838) -> ("States Out"=w837:string)  [unwired: 14 in]
      }
      frame "UI: Set String" {
        # "Set the value of the string control and indicator\nDraws from the state data and sends a public \"Value Changed\" event"
        n318 = property class="Code String LV"(reference=w854) -> (reference out=w850:refnum<class "Code String LV.lvclass">, "Properties:Text"=w848:string)  [unwired: 1 in, 1 out]
        n319 = local write "String Control"(w848) -> ()
        n320 = local write "String Indicator"(w848) -> ()
        n321 = call "Send Value Changed Event.vi"("Code String in"=w850, "Value"=w848, "error in (no error)"=w852) -> ("Code String out"=w853:refnum<class "Code String LV.lvclass">, "error out"=w851:errorcluster)  [unwired: 11 in]
        n322 = call <vilib>:"Add State(s) to Queue__jki_lib_state_machine.vi"("State(s) in (\"\")"=w857) -> ("States Out"=w856:string)  [unwired: 14 in]
      }
      frame "UI: Set Selection" {
        # "Set the text selection\n(All|Last|Start|End)"
        n323 = case shown="Default" w864 {
          selector: w864 -> [_ _ w898]
          tunnel: w866 -> [w874 w887 w899]
          tunnel: [w873 w886 w899] -> w860
          tunnel: w859 -> [w870 w884 w894]
          tunnel: [w869 w881 w895] -> w858
          frame "All" {
            n324 = property class="Code String LV"(reference=w874) -> (reference out=w873:refnum<class "Code String LV.lvclass">, "Properties:Text"=w875:string)  [unwired: 1 in, 1 out]
            n325 = String Length(string=w875) -> (length=w877:i32)
            n326 = Unbundle By Name(w870) -> ("Strings"=w872:refnum<vi>[])
            n327 = Bundle(0, w877) -> (w871:cluster{i32, i32})  [unwired: 1 in]
            n328 = for {
              tunnel: w871 -> [w880]
              tunnel: w872 -> [w879] mode=indexing
              tunnel: [w878] -> w869
              n329 = property class="Str"(reference=w879, "Text.Selection"=w880) -> (error out=w878:errorcluster)  [unwired: 1 in, 1 out]
            }
          }
          frame "Last" {
            n330 = property class="Code String LV"(reference=w887) -> (reference out=w886:refnum<class "Code String LV.lvclass">, "Properties:Text"=w888:string)  [unwired: 1 in, 1 out]
            n331 = String Length(string=w888) -> (length=w885:i32)
            n332 = Unbundle By Name(w884) -> ("Strings"=w883:refnum<vi>[])
            n333 = Bundle(w885, w885) -> (w882:cluster{i32, i32})  [unwired: 1 in]
            n334 = for {
              tunnel: w882 -> [w891]
              tunnel: w883 -> [w890] mode=indexing
              tunnel: [w889] -> w881
              n335 = property class="Str"(reference=w890, "Text.Selection"=w891) -> (error out=w889:errorcluster)  [unwired: 1 in, 1 out]
            }
          }
          frame Default {
            n336 = Scan From String(format string="%s = %d", input string=w898) -> (output 1=w892:string, output 2=w893:i32)  [unwired: 4 in, 3 out]
            n337 = Unbundle By Name(w894) -> ("Strings"=w896:refnum<vi>[])
            n338 = for {
              tunnel: w896 -> [w903] mode=indexing
              tunnel: [w902] -> w895
              tunnel: w893 -> [w901]
              tunnel: w892 -> [w900]
              n339 = case shown="\"End\"" w900 {
                tunnel: w903 -> [w906 _ w909]
                tunnel: [w905 _ w908] -> w902
                tunnel: w901 -> [w904 _ w907]
                frame "Start" {
                  n340 = property class="Str"(reference=w906, "Text.Selection Start"=w904) -> (error out=w905:errorcluster)  [unwired: 1 in, 1 out]
                }
                frame Default {
                }
                frame "End" {
                  n341 = property class="Str"(reference=w909, "Text.Selection End"=w907) -> (error out=w908:errorcluster)  [unwired: 1 in, 1 out]
                }
              }
            }
          }
        }
        n342 = property class="Code String LV"(reference=w860, error in=w858) -> (reference out=w861:refnum<class "Code String LV.lvclass">, "Properties:Active Ref"=w862:refnum<vi>)  [unwired: 1 out]
        n343 = property class="Str"(reference=w862, "Key Focus"=TRUE) -> ()  [unwired: 1 in, 2 out]
      }
      frame "UI: Set Font Size" {
        # "Update the font of both the text and the line numbers\nRetain the text selection"
        n344 = Unbundle By Name(w910) -> ("Strings"=w916:refnum<vi>[], "Line #"=w914:refnum<vi>)
        n345 = global read "Font Global.vi" "Font Size"() -> (w911:u32)
        n346 = Decrement(x=w911) -> (x-1=w913:u32)
        n347 = for {
          tunnel: w916 -> [w925] mode=indexing
          tunnel: w911 -> [w924]
          n348 = property class="Str"(reference=w925) -> (reference out=w923:refnum<vi>, "Text.Selection"=w922:T12)  [unwired: 1 in, 1 out]
          n349 = property class="Str"(reference=w923, "Text.Selection"=T7 {"Selection Start"=0, "Selection End"=-1}, "Text.FontSize"=w924, "Text.Selection"=w922) -> ()  [unwired: 1 in, 2 out]
        }
        n350 = property class="LstBox (strict)"(reference=w914, "Active Row"=-2 ("Active Row:Active Row Number"), "Cell Height"=w913, "CellFontSize"=w911) -> ()  [unwired: 1 in, 2 out]
        n351 = call <vilib>:"Add State(s) to Queue__jki_lib_state_machine.vi"("State(s) in (\"\")"=w920) -> ("States Out"=w919:string)  [unwired: 14 in]
      }
      frame "UI: Set Font Color" {
        # "Update the font color\nApplies to the current text selection"
        n352 = Decimal String To Number(string=w927, default (0L)=u32 0 ("default (0 I32)")) -> (number=w928:u32)  [unwired: 1 in, 1 out]
        n353 = Unbundle By Name(w929) -> ("Strings"=w931:refnum<vi>[])
        n354 = for {
          tunnel: w931 -> [w937] mode=indexing
          tunnel: w928 -> [w936]
          n355 = property class="Str"(reference=w937, "Text.FontColor"=w936) -> ()  [unwired: 1 in, 2 out]
        }
        n356 = call <vilib>:"Add State(s) to Queue__jki_lib_state_machine.vi"("State(s) in (\"\")"=w935) -> ("States Out"=w934:string)  [unwired: 14 in]
      }
      frame "UI: Set Selected Line Number" {
        # "Synchronize the Line Number Listbox to the current text selection\nCalled after clicking or otherwise moving the text selection cursor"
        n357 = case shown="\"\"" w946 {
          selector: w946 -> [w953 _]
          tunnel: [w952 w959] -> w945
          tunnel: w947 -> [_ w955]
          frame Default {
            n358 = Decimal String To Number(string=w953) -> (number=w952:i32)  [unwired: 2 in, 1 out]
          }
          frame "" {
            n359 = property class="Code String LV"(reference=w955) -> ("Properties:Active Ref"=w954:refnum<vi>)  [unwired: 1 in, 2 out]
            n360 = property class="Str"(reference=w954) -> ("Value"=w958:string, "Text.Selection End"=w956:u32)  [unwired: 1 in, 2 out]
            n361 = String Subset(string=w958, length (rest)=w956) -> (substring=w957:string)  [unwired: 1 in]
            n362 = case shown="Default" w957 {
              selector: w957 -> [_ w964]
              tunnel: [0 w962] -> w959
              frame "" {
              }
              frame Default {
                n363 = call "Count Lines.vi"("String"=w964, "Discard Last if Empty? (T)"=FALSE) -> ("# Lines"=w963:i32)  [unwired: 13 in]
                n364 = Decrement(x=w963) -> (x-1=w962:i32)
              }
            }
          }
        }
        n365 = Unbundle By Name(w944) -> ("Line #"=w938:refnum<vi>)
        n366 = property class="LstBox (strict)"(reference=w938) -> ("Item Names"=w939:string[])  [unwired: 1 in, 2 out]
        n367 = Array Size(array=w939) -> (size(s)=w940:i32)
        n368 = Decrement(x=w940) -> (x-1=w942:i32)
        n369 = In Range and Coerce(upper limit=w942, x=w945, lower limit=0) -> (coerced(x)=w943:i32)  [unwired: 1 out]
        n370 = local write "Line Numbers"(w943) -> ()
        n371 = call <vilib>:"Add State(s) to Queue__jki_lib_state_machine.vi"("State(s) in (\"\")"=w951) -> ("States Out"=w950:string)  [unwired: 14 in]
      }
      frame "UI: Adjust Line Numbers" {
        # "Update the Line Numbers according to the total number of lines in the String\nCalled after the String value changes"
        n372 = property class="Code String LV"(reference=w973) -> ("Properties:Text"=w974:string)  [unwired: 1 in, 2 out]
        n373 = Unbundle By Name(w967) -> ("Line #"=w965:refnum<vi>)
        n374 = Unbundle By Name(w967) -> ("Scrollbar"=w966:refnum<vi>)
        n375 = case shown="Default" w974 {
          selector: w974 -> [_ w985]
          tunnel: w965 -> [w981 w986]
          tunnel: [w980 w982] -> w972
          tunnel: [w979 w983] -> w971
          frame "" {
            w979 = 1 ("Total Number of Lines")
            # "/* Special case for empty string. We always want line 1 */"
            n376 = call "Populate Line Numbers.vi"("Line Numbers in"=w981, "Total Number of Lines"=w979) -> ("Line Numbers out"=w980:refnum<vi>)  [unwired: 13 in]
          }
          frame Default {
            # "/* Count the number of lines in the string and update the line numbers */"
            n377 = call "Count Lines.vi"("String"=w985, "Discard Last if Empty? (T)"=FALSE) -> ("# Lines"=w983:i32)  [unwired: 13 in]
            n378 = call "Populate Line Numbers.vi"("Line Numbers in"=w986, "Total Number of Lines"=w983) -> ("Line Numbers out"=w982:refnum<vi>)  [unwired: 13 in]
          }
        }
        n379 = property class="Scroll (strict)"(reference=w966) -> (reference out=w970:refnum<vi>, "PageSize"=w969:dbl)  [unwired: 1 in, 1 out]
        n380 = call "Calculate Scroll Max.vi"("ListBox Ref in"=w972, "Total Number of Lines"=w971, "Page Size"=w969) -> ("Scroll Max"=w968:i32)  [unwired: 11 in, 1 out]
        n381 = property class="Scroll (strict)"(reference=w970, "DocMax"=w968) -> ()  [unwired: 1 in, 2 out]
        n382 = call <vilib>:"Add State(s) to Queue__jki_lib_state_machine.vi"("State(s) in (\"\")"=w978) -> ("States Out"=w977:string)  [unwired: 14 in]
      }
      frame "UI: Sync Scroll" {
        # "Synchronize the scroll values of all elements\nWhen navigating the string control, we need to adjust the listbox row and the scrollbar value"
        n383 = property class="Code String LV"(reference=w995) -> ("Properties:Active Ref"=w996:refnum<vi>)  [unwired: 1 in, 2 out]
        n384 = Unbundle By Name(w992) -> ("Line #"=w991:refnum<vi>)
        n385 = case shown="Default" w997 {
          selector: w997 -> [_ w1014 _]
          tunnel: w996 -> [w1011 w1016 w1018]
          tunnel: [w1010 w1013 w1017] -> w990
          tunnel: w991 -> [w1012 _ _]
          frame "Selection" {
            n386 = call "Ensure Visible.vi"("Line Numbers"=w1012, "String in"=w1011) -> ("Scroll Position"=w1010:u32)  [unwired: 8 in, 1 out]
          }
          frame Default {
            n387 = Decimal String To Number(string=w1014) -> (number=w1015:i32)  [unwired: 2 in, 1 out]
            n388 = property class="Str"(reference=w1016, "Text.Scroll Position"=w1015) -> ("Text.Scroll Position"=w1013:u32)  [unwired: 1 in, 2 out]
          }
          frame "" {
            n389 = property class="Str"(reference=w1018) -> ("Text.Scroll Position"=w1017:u32)  [unwired: 1 in, 2 out]
          }
        }
        n390 = call-poly <userlib>:"Data Changed__ogtk.vi"("U32"=w990) -> ("Changed"=w989:bool)
        n391 = First Call?() -> (First Call?: T/F=w987:bool)
        n392 = Or(x=w989, y=w987) -> (x .or. y?=w988:bool)
        n393 = case shown="True" w988 {
          tunnel: w990 -> [_ w1005]
          tunnel: w994 -> [w1001 w1002]
          tunnel: [w1001 w1002] -> w993
          tunnel: w992 -> [_ w1004]
          frame False {
          }
          frame True {
            n394 = Unbundle By Name(w1004) -> ("Strings"=w1006:refnum<vi>[], "Scrollbar"=w1007:refnum<vi>, "Line #"=w1003:refnum<vi>)
            n395 = property class="LstBox (strict)"(reference=w1003, "Top Row"=w1005) -> ()  [unwired: 1 in, 2 out]
            n396 = for {
              tunnel: w1006 -> [w1009] mode=indexing
              tunnel: w1005 -> [w1008]
              n397 = property class="Str"(reference=w1009, "Text.Scroll Position"=w1008) -> ()  [unwired: 1 in, 2 out]
            }
            n398 = property class="Scroll (strict)"(reference=w1007, "Value"=w1005) -> ()  [unwired: 1 in, 2 out]
          }
        }
        n399 = call <vilib>:"Add State(s) to Queue__jki_lib_state_machine.vi"("State(s) in (\"\")"=w1000) -> ("States Out"=w999:string)  [unwired: 14 in]
      }
      frame "---------- Suggestions ----------" {
        # "Do not put any code in this frame.\n(It is a separator no-op. You can make a copy of this frame to create a new UI frame)"
        n400 = call <vilib>:"Add State(s) to Queue__jki_lib_state_machine.vi"("State(s) in (\"\")"=w1024) -> ("States Out"=w1023:string)  [unwired: 14 in]
      }
      frame "Suggestions: Search" {
        # "Search for Suggestions\nRead the Keywords from the dictionary and identify the position of the suggestion box"
        n401 = property class="Code String LV"(reference=w1034) -> ("Properties:Active Ref"=w1033:refnum<vi>, "Properties:Delimiter Pattern"=w1031:string, "Properties:Keywords"=w1026:string[])  [unwired: 1 in, 2 out]
        n402 = property on="Property Node" class="Str"(reference=w1033) -> ("Value"=w1030:string, "Text.Selection Start"=w1029:u32)  [unwired: 1 in, 2 out]
        n403 = call "Find Delimited String.vi"("String"=w1030, "Delimiter Regular Expression ([\\r\\n])"=w1031, "Start Offset (0)"=w1029, "End Offset (0)"=w1029) -> ("Substring"=w1027:string, "Location"=w1028:T12)  [unwired: 10 in]
        n404 = Bundle By Name(cluster=w1032, "Suggestions.Update Data.Query"=w1027, "Suggestions.Location"=w1028, "Suggestions.Update Data.Keywords"=w1026, "Suggestions.Visible?"=TRUE) -> (w1036:T14)
        n405 = call <vilib>:"Add State(s) to Queue__jki_lib_state_machine.vi"("State(s) in (\"\")"=w1039) -> ("States Out"=w1038:string)  [unwired: 14 in]
      }
      frame "Suggestions: Position" {
        # "Determine the position of the suggestion box\nCalculate based on the position of the string control and selection cursor"
        n406 = Unbundle By Name(w1041) -> ("Core.Current VI Reference"=w1040:refnum<vi>)
        n407 = property class="Code String LV"(reference=w1054) -> ("Properties:Active Ref"=w1044:refnum<vi>)  [unwired: 1 in, 2 out]
        n408 = control-ref of="Text Pane"() -> (w1048:refnum<vi>)
        n409 = call "Get Caller Coordinates.vi"("Control in"=w1044, "Pane"=w1048, "VI"=w1040, "error in (no error)"=w1046) -> ("Control out"=w1043:refnum<vi>, "Control Position"=w1047:T6, "error out"=w1045:errorcluster)  [unwired: 8 in, 1 out]
        n410 = Unbundle By Name(w1041) -> ("Suggestions.Update Data.Keywords"=w1052:string[], "Suggestions.Location"=w1050:T12, "Line #"=w1042:refnum<vi>)
        n411 = Empty Array?(array=w1052) -> (empty?=w1051:bool)
        n412 = case shown="False" w1051 {
          tunnel: w1042 -> [w1062 _]
          tunnel: [w1061 T8 {"Left"=0, "Top"=0} ("Cursor Position")] -> w1049
          tunnel: w1043 -> [w1060 _]
          tunnel: w1050 -> [w1059 _]
          tunnel: w1047 -> [w1058 _]
          frame False {
            n413 = call "Get Cursor Position.vi"("Screen Offset"=w1058, "Text Offset"=w1059, "Line Numbers in"=w1062, "String in"=w1060) -> ("Autocomplete Position"=w1061:T8)  [unwired: 7 in]
          }
          frame True {
          }
        }
        n414 = Bundle By Name(cluster=w1041, "Suggestions.Update Data.Position"=w1049) -> (w1053:T14)
        n415 = call <vilib>:"Add State(s) to Queue__jki_lib_state_machine.vi"("State(s) in (\"\")"=w1057) -> ("States Out"=w1056:string)  [unwired: 14 in]
      }
      frame "Suggestions: Decide" {
        # "Determine if the Suggestion Box should be hidden\nHide if the selected token has changed"
        n416 = Unbundle By Name(w1065) -> ("Suggestions.Delta?"=w1064:bool)
        n417 = Select(t="Suggestions: UI >> Cancel", s=w1064, f="") -> (s? t:f=w1066:string)
        n418 = call <vilib>:"Add State(s) to Queue__jki_lib_state_machine.vi"("State(s) in Front (\"\")"=w1066, "State(s) in (\"\")"=w1073) -> ("States Out"=w1072:string)  [unwired: 13 in]
      }
      frame "Suggestions: UI" {
        # "Manage the Suggestion Box UI\n(Create|Update|Next|Previous|Cancel|Accept|Destroy)"
        n419 = case shown="\"Font\"" w1076 {
          tunnel: w1081 -> [w1088 w1092 w1098 w1104 w1108 w1125 w1132 w1141 w1146]
          tunnel: [w1087 w1092 w1098 w1104 w1109 w1122 w1129 w1141 w1146] -> w1079
          tunnel: w1078 -> [w1085 w1094 w1100 w1106 w1112 w1127 w1134 w1143 w1145]
          tunnel: [w1084 w1091 w1097 w1103 w1110 w1124 w1131 w1140 w1145] -> w1077
          tunnel: w1075 -> [w1083 w1093 w1099 w1105 w1111 w1126 w1133 w1142 w1144]
          tunnel: [w1083 w1093 w1099 w1105 w1111 w1126 w1133 w1142 w1144] -> w1074
          frame "Create" {
            n420 = call "Create Suggestion Box.vi"("error in (no error)"=w1085) -> ("Suggestion Box out"=w1086:refnum<class "Suggestion Box.lvclass">, "error out"=w1084:errorcluster)  [unwired: 13 in]
            n421 = Bundle By Name(cluster=w1088, "Suggestions.Suggestion Box"=w1086) -> (w1087:T14)
          }
          frame "Update" {
            n422 = Unbundle By Name(w1092) -> ("Suggestions.Suggestion Box"=w1090:refnum<class "Suggestion Box.lvclass">, "Suggestions.Update Data"=w1089:T11)
            n423 = call "Display Suggestion Box.vi"("Suggestion Box in"=w1090, "Update Data"=w1089, "error in (no error)"=w1094) -> ("error out"=w1091:errorcluster)  [unwired: 11 in, 1 out]
          }
          frame "Next" {
            n424 = Unbundle By Name(w1098) -> ("Suggestions.Suggestion Box"=w1096:refnum<class "Suggestion Box.lvclass">)
            n425 = call "Navigate Suggestions.vi"("Suggestion Box in"=w1096, "Next?"=TRUE, "error in (no error)"=w1100) -> ("error out"=w1097:errorcluster)  [unwired: 11 in, 1 out]
          }
          frame "Previous" {
            n426 = Unbundle By Name(w1104) -> ("Suggestions.Suggestion Box"=w1102:refnum<class "Suggestion Box.lvclass">)
            n427 = call "Navigate Suggestions.vi"("Suggestion Box in"=w1102, "Next?"=FALSE, "error in (no error)"=w1106) -> ("error out"=w1103:errorcluster)  [unwired: 11 in, 1 out]
          }
          frame "Cancel" {
            n428 = Unbundle By Name(w1108) -> ("Suggestions.Visible?"=w1107:bool)
            n429 = case shown="True" w1107 {
              tunnel: w1112 -> [w1113 w1120]
              tunnel: w1108 -> [w1114 w1119]
              tunnel: [w1113 w1118] -> w1110
              tunnel: [w1114 w1116] -> w1109
              frame False {
              }
              frame True {
                n430 = Unbundle By Name(w1119) -> ("Suggestions.Suggestion Box"=w1117:refnum<class "Suggestion Box.lvclass">)
                n431 = Bundle By Name(cluster=w1119, "Suggestions.Visible?"=FALSE ("Suggestions.Available?")) -> (w1116:T14)
                n432 = call "Cancel Suggestion.vi"("Suggestion Box in"=w1117, "error in (no error)"=w1120) -> ("error out"=w1118:errorcluster)  [unwired: 12 in, 1 out]
              }
            }
          }
          frame "Accept" {
            n433 = Unbundle By Name(w1125) -> ("Suggestions.Suggestion Box"=w1123:refnum<class "Suggestion Box.lvclass">)
            n434 = Bundle By Name(cluster=w1125, "Suggestions.Visible?"=FALSE) -> (w1122:T14)
            n435 = call "Accept Suggestion.vi"("Suggestion Box in"=w1123, "error in (no error)"=w1127) -> ("error out"=w1124:errorcluster)  [unwired: 12 in, 1 out]
          }
          frame "Destroy" {
            n436 = Unbundle By Name(w1132) -> ("Suggestions.Suggestion Box"=w1130:refnum<class "Suggestion Box.lvclass">)
            n437 = Bundle By Name(cluster=w1132, "Suggestions.Visible?"=FALSE) -> (w1129:T14)
            n438 = call "Destroy Suggestion Box.vi"("Suggestion Box in"=w1130, "error in (no error)"=w1134) -> ("error out"=w1131:errorcluster)  [unwired: 12 in, 1 out]
          }
          frame "Font" {
            n439 = Unbundle By Name(w1141) -> ("Suggestions.Suggestion Box"=w1139:refnum<class "Suggestion Box.lvclass">)
            n440 = global read "Font Global.vi" "Font Size"() -> (w1137:u32)
            n441 = global read "Font Global.vi" "Font"() -> (w1135:string)
            n442 = Bundle By Name(cluster=T9 {"Font Name"="Consolas", "Size"=14, "Bold"=FALSE, "Italic"=FALSE, "Underline"=FALSE, "Strikeout"=FALSE, "Color"=7171459} ("Font"), "Size"=w1137, "Font Name"=w1135) -> (w1136:T9)
            n443 = call "Set Font.vi"("Suggestion Box in"=w1139, "Font"=w1136, "error in (no error)"=w1143) -> ("error out"=w1140:errorcluster)  [unwired: 11 in, 1 out]
          }
          frame Default {
          }
        }
      }
      frame "---------- Macro ----------" {
        # "Do not put any code in this frame.\n(It is a separator no-op. You can make a copy of this frame to create a new Macro frame)"
        n444 = call <vilib>:"Add State(s) to Queue__jki_lib_state_machine.vi"("State(s) in (\"\")"=w1152) -> ("States Out"=w1151:string)  [unwired: 14 in]
      }
      frame "Macro: Initialize" {
        # "Initialization Macro\n(This is called once, when the VI starts)"
        n445 = call <vilib>:"Add State(s) to Queue__jki_lib_state_machine.vi"("State(s) in Front (\"\")"="Data: Initialize\nInitialize Core Data\nUI: Set Active Ref\nUI: Initialize\nSuggestions: UI >> Create\nData: Register Events\nUI: Resize\nUI: Sync Scroll\nProcess Sync", "State(s) in (\"\")"=w1159) -> ("States Out"=w1158:string)  [unwired: 13 in]
      }
      frame "Macro: Process Text" {
        # "Process state text\nUpdate selection, line numbers, and navigation"
        n446 = property class="Code String LV"(reference=w1170) -> ("Properties:Text"=w1168:string)  [unwired: 1 in, 2 out]
        n447 = call "Count Lines.vi"("String"=w1168, "Discard Last if Empty? (T)"=FALSE) -> ("# Lines"=w1167:i32)  [unwired: 13 in]
        n448 = call-poly <userlib>:"Data Changed__ogtk.vi"("I32"=w1167) -> ("Changed"=w1162:bool)
        n449 = First Call?() -> (First Call?: T/F=w1160:bool)
        n450 = Or(x=w1162, y=w1160) -> (x .or. y?=w1161:bool)
        n451 = case shown="True" w1161 {
          tunnel: [_ "UI: Adjust Line Numbers\nMacro: Navigate Lines"] -> w1164
          frame False {
          }
          frame True {
          }
        }
        n452 = case shown="\"Move Cursor\"" w1172 {
          tunnel: [_ "UI: Set Selection >> Last"] -> w1173
          frame Default {
          }
          frame "Move Cursor" {
          }
        }
        n453 = call <vilib>:"Add State(s) to Queue__jki_lib_state_machine.vi"("State(s) in Front (\"\")"="Data: Update Selection", "State(s) in (\"\")"=w1164, "State(s) at Back (\"\")"="UI: Defer Updates >> False") -> ("States Out"=w1163:string)  [unwired: 12 in]
        n454 = call <vilib>:"Add State(s) to Queue__jki_lib_state_machine.vi"("State(s) in Front (\"\")"="UI: Defer Updates >> True\nUI: Set String", "State(s) in (\"\")"=w1173, "State(s) at Back (\"\")"=w1163) -> ("States Out"=w1174:string)  [unwired: 12 in]
        n455 = call <vilib>:"Add State(s) to Queue__jki_lib_state_machine.vi"("State(s) in Front (\"\")"=w1174, "State(s) in (\"\")"=w1179) -> ("States Out"=w1178:string)  [unwired: 13 in]
      }
      frame "Macro: Handle Text Entry" {
        # "Respond to text entry\nUpdate line numbers and navigation and optionally display the suggestions box"
        n456 = call <vilib>:"Build State String with Arguments__jki_lib_state_machine.vi"("Arguments (\"\")"=w1183, "State"="Macro: Process Text") -> ("State with Arguments"=w1182:string)  [unwired: 4 in]
        n457 = call <vilib>:"Add State(s) to Queue__jki_lib_state_machine.vi"("State(s) in Front (\"\")"="Data: Set String State", "State(s) at Back (\"\")"=w1182) -> ("States Out"=w1186:string)  [unwired: 13 in]
        n458 = call <vilib>:"Add State(s) to Queue__jki_lib_state_machine.vi"("State(s) in Front (\"\")"=w1186, "State(s) in (\"\")"=w1192) -> ("States Out"=w1191:string)  [unwired: 13 in]
      }
      frame "Macro: Handle Suggestions" {
        # "Handle suggestions\nSearch and (if matches found) display the suggestion box"
        n459 = call <vilib>:"Add State(s) to Queue__jki_lib_state_machine.vi"("State(s) in Front (\"\")"="Suggestions: Search\nSuggestions: Position\nSuggestions: UI >> Update", "State(s) in (\"\")"=w1199) -> ("States Out"=w1198:string)  [unwired: 13 in]
      }
      frame "Macro: Select All" {
        # "Select all of the text in the Code String\ne.g. via CTRL+A or shortcut menu"
        n460 = call <vilib>:"Add State(s) to Queue__jki_lib_state_machine.vi"("State(s) in Front (\"\")"="UI: Set Selection >> All\nData: Update Selection", "State(s) in (\"\")"=w1206) -> ("States Out"=w1205:string)  [unwired: 13 in]
      }
      frame "Macro: Navigate Lines" {
        # "Navigate line-by-line\nUpdate line numbers and scroll position"
        n461 = Empty String/Path?(string/path=w1207) -> (empty?=w1212:bool)
        n462 = Select(t="UI: Defer Updates >> True", s=w1212, f="") -> (s? t:f=w1210:string)
        n463 = Select(t="UI: Defer Updates >> False", s=w1212, f="") -> (s? t:f=w1209:string)
        n464 = call <vilib>:"Add State(s) to Queue__jki_lib_state_machine.vi"("State(s) in Front (\"\")"=w1210, "State(s) in (\"\")"="UI: Set Selected Line Number\nUI: Sync Scroll >> Selection", "State(s) at Back (\"\")"=w1209) -> ("States Out"=w1208:string)  [unwired: 12 in]
        n465 = call <vilib>:"Add State(s) to Queue__jki_lib_state_machine.vi"("State(s) in Front (\"\")"=w1208, "State(s) in (\"\")"=w1217) -> ("States Out"=w1222:string)  [unwired: 13 in]
      }
      frame "Macro: Sync Scroll" {
        # "Navigate line-by-line\nUpdate line numbers and scroll position"
        n466 = Empty String/Path?(string/path=w1226) -> (empty?=w1230:bool)
        n467 = Select(t="UI: Defer Updates >> True", s=w1230, f="") -> (s? t:f=w1229:string)
        n468 = Select(t="UI: Defer Updates >> False", s=w1230, f="") -> (s? t:f=w1228:string)
        n469 = call <vilib>:"Build State String with Arguments__JKI_lib_State_Machine.vi"("Arguments (\"\")"=w1224, "State"="UI: Sync Scroll") -> ("State with Arguments"=w1223:string)  [unwired: 4 in]
        n470 = call <vilib>:"Add State(s) to Queue__jki_lib_state_machine.vi"("State(s) in Front (\"\")"=w1229, "State(s) in (\"\")"=w1223, "State(s) at Back (\"\")"=w1228) -> ("States Out"=w1227:string)  [unwired: 12 in]
        n471 = call <vilib>:"Add State(s) to Queue__jki_lib_state_machine.vi"("State(s) in Front (\"\")"=w1227, "State(s) in (\"\")"=w1235) -> ("States Out"=w1240:string)  [unwired: 13 in]
      }
      frame "Macro: Exit" {
        # "Exit Macro\n(This is called once, when the VI exits)"
        n472 = Unbundle By Name(w1253) -> ("Core.Close Panel on Exit?"=w1252:bool)
        n473 = case shown="\"Sync\"" w1242 {
          tunnel: [_ "Process Sync"] -> w1241
          frame Default {
          }
          frame "Sync" {
          }
        }
        n474 = call <vilib>:"Add State(s) to Queue__jki_lib_state_machine.vi"("State(s) in Front (\"\")"="UI: Defer Updates >> True\nUI: Initialize\nSuggestions: UI >> Destroy\nData: Cleanup", "State(s) in (\"\")"=w1241, "State(s) at Back (\"\")"="UI: Defer Updates >> False\nExit") -> ("States Out"=w1243:string)  [unwired: 12 in]
        n475 = Select(t="UI: Front Panel State >> Close", s=w1252, f="") -> (s? t:f=w1249:string)
        n476 = call <vilib>:"Add State(s) to Queue__jki_lib_state_machine.vi"("State(s) in (\"\")"=w1249, "State(s) at Back (\"\")"=w1243) -> ("States Out"=w1248:string)  [unwired: 13 in]
        n477 = call <vilib>:"Add State(s) to Queue__jki_lib_state_machine.vi"("State(s) in Front (\"\")"=w1248, "State(s) in (\"\")"=w1256) -> ("States Out"=w1255:string)  [unwired: 13 in]
      }
    }
  }
